vi "clearOrCalcAllPhaseWaveforms_v02.vi"(6 "How Many Experimental Phases?":i32=10 min=1 max=14, 7 "Clear Waveform?":bool, 8 "error in":errorcluster, 9 "Waveform Simulation Jump Filter (Hz)":dbl=100.0, 10 "Waveform Simulation sampling rate (Hz)":i32=1000, 11 "ExperimentOptionsCluster":T1) -> (0 "error out":errorcluster)   [LabVIEW 2019]
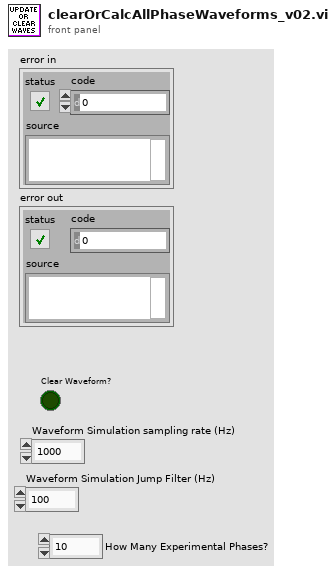
[diagram p1: front panel]
types:
  T1 = cluster{"How Many Experimental Phases?":refnum<vi>, "PhaseA Cluster":cluster{"Phase Experiment Option":refnum<vi>, "Paired Pulse":refnum<vi>, "Jump Train":refnum<vi>, "Voltage Ramp":refnum<vi>, "Voltage Step":refnum<vi>, "Solution Change":refnum<vi>, "Single Jump":refnum<vi>, "Single Manip Jump":refnum<vi>, "Gap Free":refnum<vi>, "Multi Manip Jump":refnum<vi>, "Voltage Pulse":refnum<vi>, "Current Pulse":refnum<vi>, "Current Ramp":refnum<vi>, "Gap Free Iclamp":refnum<vi>}, "PhaseB Cluster":cluster{"Phase Experiment Option":refnum<vi>, "Paired Pulse":refnum<vi>, "Jump Train":refnum<vi>, "Voltage Ramp":refnum<vi>, "Voltage Step":refnum<vi>, "Solution Change":refnum<vi>, "Single Jump":refnum<vi>, "Single Manip Jump":refnum<vi>, "Gap Free":refnum<vi>, "Multi Manip Jump":refnum<vi>, "Voltage Pulse":refnum<vi>, "Current Pulse":refnum<vi>, "Current Ramp":refnum<vi>, "Gap Free Iclamp":refnum<vi>}, "PhaseC Cluster":cluster{"Phase Experiment Option":refnum<vi>, "Paired Pulse":refnum<vi>, "Jump Train":refnum<vi>, "Voltage Ramp":refnum<vi>, "Voltage Step":refnum<vi>, "Solution Change":refnum<vi>, "Single Jump":refnum<vi>, "Single Manip Jump":refnum<vi>, "Gap Free":refnum<vi>, "Multi Manip Jump":refnum<vi>, "Voltage Pulse":refnum<vi>, "Current Pulse":refnum<vi>, "Current Ramp":refnum<vi>, "Gap Free Iclamp":refnum<vi>}, "PhaseD Cluster":cluster{"Phase Experiment Option":refnum<vi>, "Paired Pulse":refnum<vi>, "Jump Train":refnum<vi>, "Voltage Ramp":refnum<vi>, "Voltage Step":refnum<vi>, "Solution Change":refnum<vi>, "Single Jump":refnum<vi>, "Single Manip Jump":refnum<vi>, "Gap Free":refnum<vi>, "Multi Manip Jump":refnum<vi>, "Voltage Pulse":refnum<vi>, "Current Pulse":refnum<vi>, "Current Ramp":refnum<vi>, "Gap Free Iclamp":refnum<vi>}, "PhaseE Cluster":cluster{"Phase Experiment Option":refnum<vi>, "Paired Pulse":refnum<vi>, "Jump Train":refnum<vi>, "Voltage Ramp":refnum<vi>, "Voltage Step":refnum<vi>, "Solution Change":refnum<vi>, "Single Jump":refnum<vi>, "Single Manip Jump":refnum<vi>, "Gap Free":refnum<vi>, "Multi Manip Jump":refnum<vi>, "Voltage Pulse":refnum<vi>, "Current Pulse":refnum<vi>, "Current Ramp":refnum<vi>, "Gap Free Iclamp":refnum<vi>}, "PhaseF Cluster":cluster{"Phase Experiment Option":refnum<vi>, "Paired Pulse":refnum<vi>, "Jump Train":refnum<vi>, "Voltage Ramp":refnum<vi>, "Voltage Step":refnum<vi>, "Solution Change":refnum<vi>, "Single Jump":refnum<vi>, "Single Manip Jump":refnum<vi>, "Gap Free":refnum<vi>, "Multi Manip Jump":refnum<vi>, "Voltage Pulse":refnum<vi>, "Current Pulse":refnum<vi>, "Current Ramp":refnum<vi>, "Gap Free Iclamp":refnum<vi>}, "time to wait for solution change (min)":refnum<vi>, "valve Time Cluster":cluster{"time of Last V1 Change":refnum<vi>, "time of Last V2 Change":refnum<vi>, "time of Last V3 Change":refnum<vi>}, "PhaseG Cluster":cluster{"Phase Experiment Option":refnum<vi>, "Paired Pulse":refnum<vi>, "Jump Train":refnum<vi>, "Voltage Ramp":refnum<vi>, "Voltage Step":refnum<vi>, "Solution Change":refnum<vi>, "Single Jump":refnum<vi>, "Single Manip Jump":refnum<vi>, "Gap Free":refnum<vi>, "Multi Manip Jump":refnum<vi>, "Voltage Pulse":refnum<vi>, "Current Pulse":refnum<vi>, "Current Ramp":refnum<vi>, "Gap Free Iclamp":refnum<vi>}, "PhaseH Cluster":cluster{"Phase Experiment Option":refnum<vi>, "Paired Pulse":refnum<vi>, "Jump Train":refnum<vi>, "Voltage Ramp":refnum<vi>, "Voltage Step":refnum<vi>, "Solution Change":refnum<vi>, "Single Jump":refnum<vi>, "Single Manip Jump":refnum<vi>, "Gap Free":refnum<vi>, "Multi Manip Jump":refnum<vi>, "Voltage Pulse":refnum<vi>, "Current Pulse":refnum<vi>, "Current Ramp":refnum<vi>, "Gap Free Iclamp":refnum<vi>}, "PhaseI Cluster":cluster{"Phase Experiment Option":refnum<vi>, "Paired Pulse":refnum<vi>, "Jump Train":refnum<vi>, "Voltage Ramp":refnum<vi>, "Voltage Step":refnum<vi>, "Solution Change":refnum<vi>, "Single Jump":refnum<vi>, "Single Manip Jump":refnum<vi>, "Gap Free":refnum<vi>, "Multi Manip Jump":refnum<vi>, "Voltage Pulse":refnum<vi>, "Current Pulse":refnum<vi>, "Current Ramp":refnum<vi>, "Gap Free Iclamp":refnum<vi>}, "PhaseJ Cluster":cluster{"Phase Experiment Option":refnum<vi>, "Paired Pulse":refnum<vi>, "Jump Train":refnum<vi>, "Voltage Ramp":refnum<vi>, "Voltage Step":refnum<vi>, "Solution Change":refnum<vi>, "Single Jump":refnum<vi>, "Single Manip Jump":refnum<vi>, "Gap Free":refnum<vi>, "Multi Manip Jump":refnum<vi>, "Voltage Pulse":refnum<vi>, "Current Pulse":refnum<vi>, "Current Ramp":refnum<vi>, "Gap Free Iclamp":refnum<vi>}, "PhaseK Cluster":cluster{"Phase Experiment Option":refnum<vi>, "Paired Pulse":refnum<vi>, "Jump Train":refnum<vi>, "Voltage Ramp":refnum<vi>, "Voltage Step":refnum<vi>, "Solution Change":refnum<vi>, "Single Jump":refnum<vi>, "Single Manip Jump":refnum<vi>, "Gap Free":refnum<vi>, "Multi Manip Jump":refnum<vi>, "Voltage Pulse":refnum<vi>, "Current Pulse":refnum<vi>, "Current Ramp":refnum<vi>, "Gap Free Iclamp":refnum<vi>}, "PhaseL Cluster":cluster{"Phase Experiment Option":refnum<vi>, "Paired Pulse":refnum<vi>, "Jump Train":refnum<vi>, "Voltage Ramp":refnum<vi>, "Voltage Step":refnum<vi>, "Solution Change":refnum<vi>, "Single Jump":refnum<vi>, "Single Manip Jump":refnum<vi>, "Gap Free":refnum<vi>, "Multi Manip Jump":refnum<vi>, "Voltage Pulse":refnum<vi>, "Current Pulse":refnum<vi>, "Current Ramp":refnum<vi>, "Gap Free Iclamp":refnum<vi>}, "PhaseStatusCluster":cluster{"Phase A Done":refnum<vi>, "Phase B Done":refnum<vi>, "Phase C Done":refnum<vi>, "Phase D Done":refnum<vi>, "Phase E Done":refnum<vi>, "Phase F Done":refnum<vi>, "Phase G Done":refnum<vi>, "Phase H Done":refnum<vi>, "Phase I Done":refnum<vi>, "Phase J Done":refnum<vi>, "Phase K Done":refnum<vi>, "Phase L Done":refnum<vi>}}
  T2 = cluster{"Phase Experiment Option":refnum<vi>, "Paired Pulse":refnum<vi>, "Jump Train":refnum<vi>, "Voltage Ramp":refnum<vi>, "Voltage Step":refnum<vi>, "Solution Change":refnum<vi>, "Single Jump":refnum<vi>, "Single Manip Jump":refnum<vi>, "Gap Free":refnum<vi>, "Multi Manip Jump":refnum<vi>, "Voltage Pulse":refnum<vi>, "Current Pulse":refnum<vi>, "Current Ramp":refnum<vi>, "Gap Free Iclamp":refnum<vi>}
  T3 = cluster{"Which Position to use for Experiment":enum16{"Jumper Safe Position", "Experiment Safe Position", "Jumper Position A", "Jumper Position B", "Jumper Position C", "Jumper Position o-A", "Jumper Position A-o", "Jumper Position A-B", "Jumper Position B-A", "Jumper Position B-C", "Jumper Position C-B", "Jumper Position C-o", "Jumper Position o-C", "Don't Move"}, "Start Position (N)":string, "Jump Position (m)":string, "Duration (s)":dbl, "Delay (s)":dbl, "Pulse Width (s)":dbl, "Replicates":dbl, "Pulse Delay (s)":dbl, "Pulse Delta Delay (s)":dbl, "Vholding (mV)":dbl, "Valve 1 Position":i16, "Valve 2 Position":i16, "valve 1 used now?":bool, "valve 2 used now?":bool, "valve 3 used now? ":bool, "Valve 3 Position":i16, "protocol Preview":waveform(dbl)[]}
  T4 = cluster{"Which Position to use for Experiment":enum16{"Jumper Safe Position", "Experiment Safe Position", "Jumper Position A", "Jumper Position B", "Jumper Position C", "Jumper Position o-A", "Jumper Position A-o", "Jumper Position A-B", "Jumper Position B-A", "Jumper Position B-C", "Jumper Position C-B", "Jumper Position C-o", "Jumper Position o-C", "Don't Move"}, "Start Position (N)":string, "Jump Position (m)":string, "Duration (s)":dbl, "Delay (s)":dbl, "Pulse Width (s)":dbl, "Valve 1 Position":i16, "Valve 2 Position":i16, "Replicates":dbl, "Pulse Period (s)":dbl, "Vholding (mV)":dbl, "Number of Pulses":dbl, "valve 1 used now?":bool, "valve 2 used now?":bool, "valve 3 used now? ":bool, "Valve 3 Position":i16, "protocol Preview":waveform(dbl)[]}
  T5 = cluster{"Which Position to use for Experiment":enum16{"Jumper Safe Position", "Experiment Safe Position", "Jumper Position A", "Jumper Position B", "Jumper Position C", "Jumper Position o-A", "Jumper Position A-o", "Jumper Position A-B", "Jumper Position B-A", "Jumper Position B-C", "Jumper Position C-B", "Jumper Position C-o", "Jumper Position o-C", "Don't Move"}, "Duration (s)":dbl, "Delay (s)":dbl, "Ramp Slope (mV/s)":dbl, "Voltage Start (mV)":dbl, "Replicates":dbl, "Voltage End (mV)":dbl, "Ramp Duration (s)":dbl, "Vholding (mV)":dbl, "Valve 1 Position":i16, "Valve 2 Position":i16, "Valve 3 Position":i16, "valve 1 used now?":bool, "valve 2 used now?":bool, "valve 3 used now? ":bool, "Maintain Final Voltage until end?":bool, "protocol Preview":waveform(dbl)[]}
  T6 = cluster{"Which Position to use for Experiment":enum16{"Jumper Safe Position", "Experiment Safe Position", "Jumper Position A", "Jumper Position B", "Jumper Position C", "Jumper Position o-A", "Jumper Position A-o", "Jumper Position A-B", "Jumper Position B-A", "Jumper Position B-C", "Jumper Position C-B", "Jumper Position C-o", "Jumper Position o-C", "Don't Move"}, "Duration (s)":dbl, "Delay (s)":dbl, "Ramp Slope (pA/s)":dbl, "Current Start (pA)":dbl, "Replicates":dbl, "Current End (pA)":dbl, "Ramp Duration (s)":dbl, "Iholding (pA)":dbl, "Valve 1 Position":i16, "Valve 2 Position":i16, "Valve 3 Position":i16, "valve 1 used now?":bool, "valve 2 used now?":bool, "valve 3 used now? ":bool, "Maintain Final Voltage until end?":bool, "protocol Preview":waveform(dbl)[]}
  T7 = cluster{"Which Position to use for Experiment":enum16{"Jumper Safe Position", "Experiment Safe Position", "Jumper Position A", "Jumper Position B", "Jumper Position C", "Jumper Position o-A", "Jumper Position A-o", "Jumper Position A-B", "Jumper Position B-A", "Jumper Position B-C", "Jumper Position C-B", "Jumper Position C-o", "Jumper Position o-C", "Don't Move"}, "Duration (s)":dbl, "Delay (s)":dbl, "Step Width (s)":dbl, "Voltage Start (mV)":dbl, "Voltage Step (mV)":dbl, "Replicates":dbl, "Voltage End (mV)":dbl, "Number of Step":dbl, "Vholding (mV)":dbl, "Valve 1 Position":i16, "Valve 2 Position":i16, "Valve 3 Position":i16, "valve 1 used now?":bool, "valve 2 used now?":bool, "valve 3 used now? ":bool, "Total Step Time (s)":dbl, "Maintain Final Voltage until end?":bool, "protocol Preview":waveform(dbl)[]}
  T8 = cluster{"Which Position to use for Experiment":enum16{"Jumper Safe Position", "Experiment Safe Position", "Jumper Position A", "Jumper Position B", "Jumper Position C", "Jumper Position o-A", "Jumper Position A-o", "Jumper Position A-B", "Jumper Position B-A", "Jumper Position B-C", "Jumper Position C-B", "Jumper Position C-o", "Jumper Position o-C", "Don't Move"}, "Duration (s)":dbl, "Delay (s)":dbl, "Pulse Width (s)":dbl, "Which Valve to Change?":i16, "Valve Jump Position":i16, "Replicates":dbl, "Vholding (mV)":dbl, "valve 1 used now?":bool, "valve 2 used now?":bool, "valve 3 used now? ":bool, "Valve 1 Position":i16, "Valve 2 Position":i16, "Valve 3 Position":i16, "protocol Preview":waveform(dbl)[]}
  T9 = cluster{"Which Position to use for Experiment":enum16{"Jumper Safe Position", "Experiment Safe Position", "Jumper Position A", "Jumper Position B", "Jumper Position C", "Jumper Position o-A", "Jumper Position A-o", "Jumper Position A-B", "Jumper Position B-A", "Jumper Position B-C", "Jumper Position C-B", "Jumper Position C-o", "Jumper Position o-C", "Don't Move"}, "Start Position (N)":string, "Jump Position (m)":string, "Duration (s)":dbl, "Delay (s)":dbl, "Pulse Width (s)":dbl, "Valve 1 Position":i16, "Valve 2 Position":i16, "Replicates":dbl, "Vholding (mV)":dbl, "Valve 3 Position":i16, "valve 1 used now?":bool, "valve 2 used now?":bool, "valve 3 used now? ":bool, "protocol Preview":waveform(dbl)[]}
  T10 = cluster{"Start Position (N)":enum16{"Jumper Safe Position", "Experiment Safe Position", "Jumper Position A", "Jumper Position B", "Jumper Position C", "Jumper Position o-A", "Jumper Position A-o", "Jumper Position A-B", "Jumper Position B-A", "Jumper Position B-C", "Jumper Position C-B", "Jumper Position C-o", "Jumper Position o-C", "Don't Move"}, "Duration (s)":dbl, "Delay (s)":dbl, "Pulse Width (s)":dbl, "Valve 1 Position":i16, "Valve 2 Position":i16, "Replicates":dbl, "Jump Position (m)":enum16{"Jumper Safe Position", "Experiment Safe Position", "Jumper Position A", "Jumper Position B", "Jumper Position C", "Jumper Position o-A", "Jumper Position A-o", "Jumper Position A-B", "Jumper Position B-A", "Jumper Position B-C", "Jumper Position C-B", "Jumper Position C-o", "Jumper Position o-C", "Don't Move"}, "Vholding (mV)":dbl, "Valve 3 Position":i16, "valve 1 used now?":bool, "valve 2 used now?":bool, "valve 3 used now? ":bool, "protocol Preview":waveform(dbl)[]}
  T11 = cluster{"Start Position (N)":enum16{"Jumper Safe Position", "Experiment Safe Position", "Jumper Position A", "Jumper Position B", "Jumper Position C", "Jumper Position o-A", "Jumper Position A-o", "Jumper Position A-B", "Jumper Position B-A", "Jumper Position B-C", "Jumper Position C-B", "Jumper Position C-o", "Jumper Position o-C"}, "Duration (s)":dbl, "Delay (s)":dbl, "Valve 1 Position":i16, "Valve 2 Position":i16, "Replicates":dbl, "Vholding (mV)":dbl, "Valve 3 Position":i16, "valve 1 used now?":bool, "valve 2 used now?":bool, "valve 3 used now? ":bool, "Jump Position Array":enum16{"Jumper Safe Position", "Experiment Safe Position", "Jumper Position A", "Jumper Position B", "Jumper Position C", "Jumper Position o-A", "Jumper Position A-o", "Jumper Position A-B", "Jumper Position B-A", "Jumper Position B-C", "Jumper Position C-B", "Jumper Position C-o", "Jumper Position o-C"}[], "Position Dwell Time (s)":dbl[], "protocol Preview":waveform(dbl)[]}
  T12 = cluster{"Which Position to use for Experiment":enum16{"Jumper Safe Position", "Experiment Safe Position", "Jumper Position A", "Jumper Position B", "Jumper Position C", "Jumper Position o-A", "Jumper Position A-o", "Jumper Position A-B", "Jumper Position B-A", "Jumper Position B-C", "Jumper Position C-B", "Jumper Position C-o", "Jumper Position o-C", "Don't Move"}, "Duration (s)":dbl, "Delay (s)":dbl, "Pulse 2 (s)":dbl, "Pulse 1 (mV)":dbl, "Replicates":dbl, "Pulse 1 (s)":dbl, "Pulse 2 (mV)":dbl, "Vholding (mV)":dbl, "Valve 1 Position":i16, "Valve 2 Position":i16, "Valve 3 Position":i16, "valve 1 used now?":bool, "valve 2 used now?":bool, "valve 3 used now? ":bool, "Maintain Final Voltage until end?":bool, "delta Pulse 1 (mV)":dbl, "delta Pulse 2 (mV)":dbl, "Sweeps":dbl, "Final Pulse 1 (mV)":dbl, "Final Pulse 2 (mV)":dbl, "protocol Preview":waveform(dbl)[]}
  T13 = cluster{"Which Position to use for Experiment":enum16{"Jumper Safe Position", "Experiment Safe Position", "Jumper Position A", "Jumper Position B", "Jumper Position C", "Jumper Position o-A", "Jumper Position A-o", "Jumper Position A-B", "Jumper Position B-A", "Jumper Position B-C", "Jumper Position C-B", "Jumper Position C-o", "Jumper Position o-C", "Don't Move"}, "Duration (s)":dbl, "Delay (s)":dbl, "Pulse 2 (s)":dbl, "Pulse 1 (pA)":dbl, "Replicates":dbl, "Pulse 1 (s)":dbl, "Pulse 2 (pA)":dbl, "Iholding (pA)":dbl, "Valve 1 Position":i16, "Valve 2 Position":i16, "Valve 3 Position":i16, "valve 1 used now?":bool, "valve 2 used now?":bool, "valve 3 used now? ":bool, "Maintain Final Voltage until end?":bool, "delta Pulse 1 (pA)":dbl, "delta Pulse 2 (pA)":dbl, "Sweeps":dbl, "Final Pulse 1 (pA)":dbl, "Final Pulse 2 (pA)":dbl, "protocol Preview":waveform(dbl)[]}
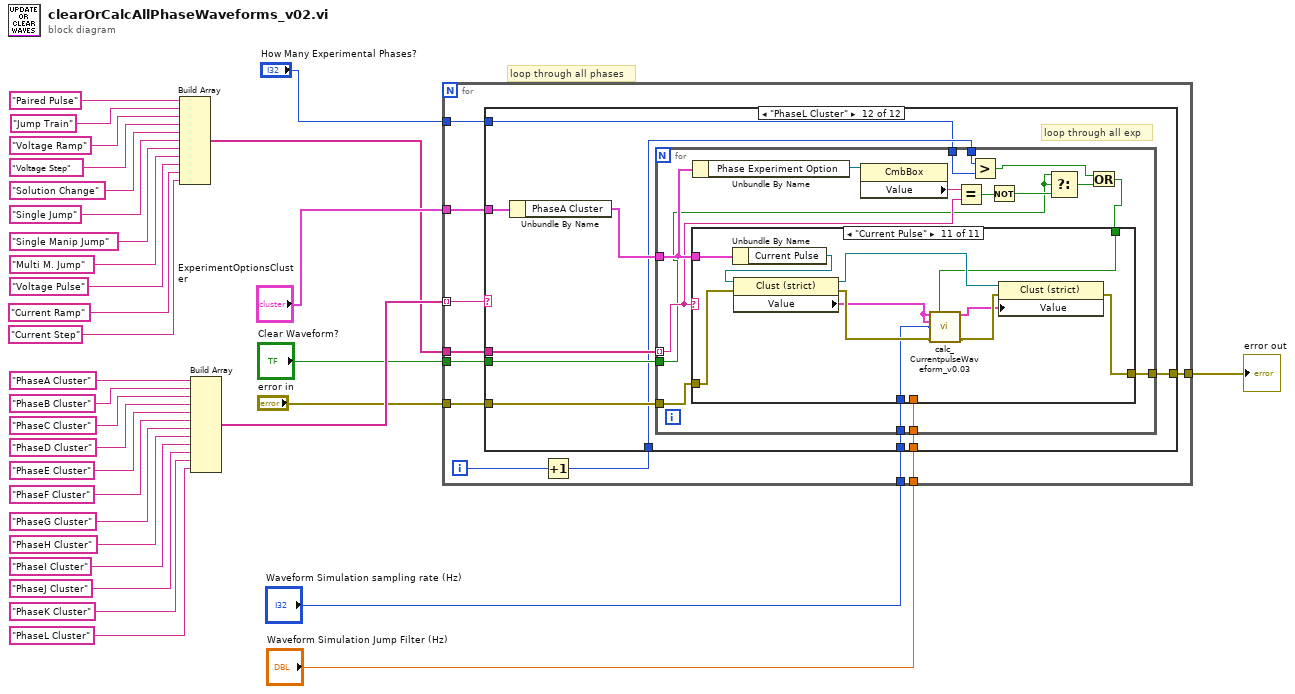
[diagram p0: block diagram]
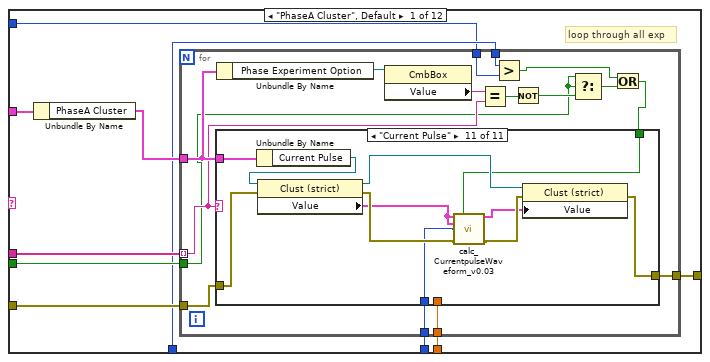
[diagram p2: hidden frame]
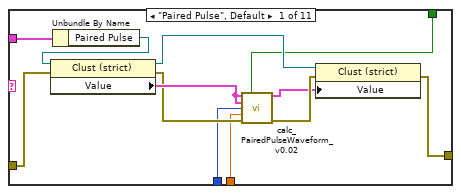
[diagram p3: hidden frame]
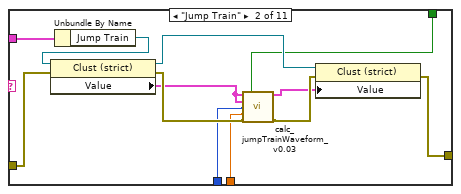
[diagram p4: hidden frame]
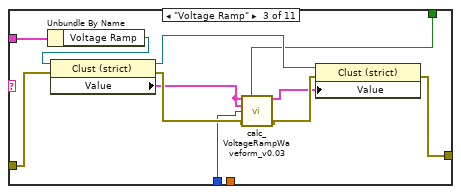
[diagram p5: hidden frame]
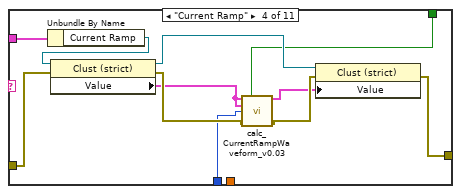
[diagram p6: hidden frame]
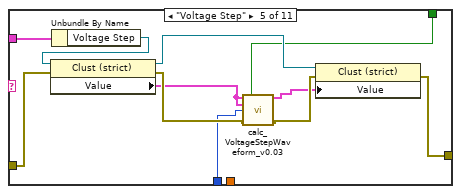
[diagram p7: hidden frame]
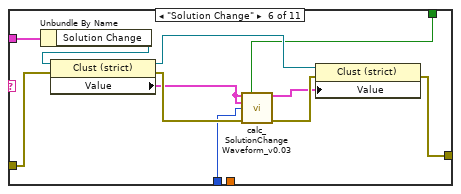
[diagram p8: hidden frame]
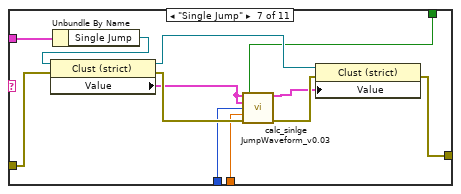
[diagram p9: hidden frame]
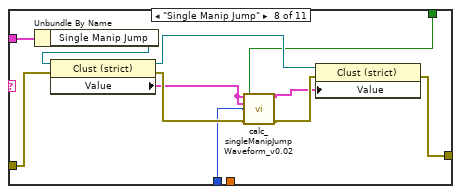
[diagram p10: hidden frame]
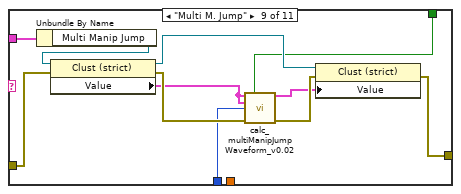
[diagram p11: hidden frame]
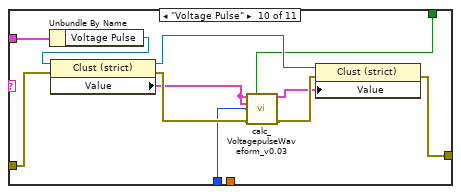
[diagram p12: hidden frame]
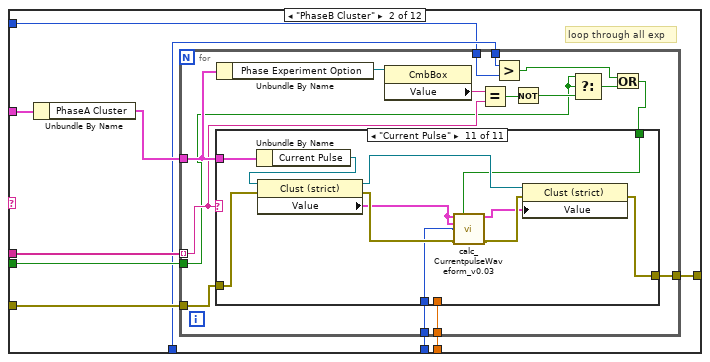
[diagram p13: hidden frame]
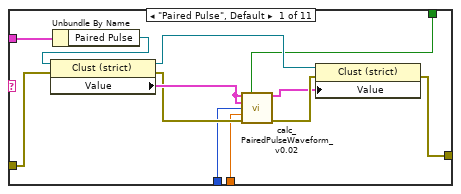
[diagram p14: hidden frame]
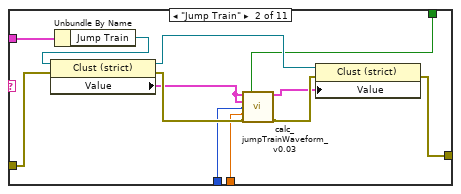
[diagram p15: hidden frame]
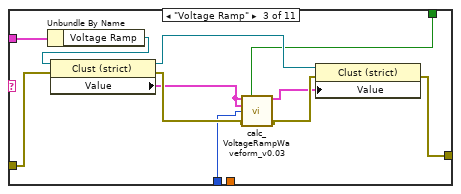
[diagram p16: hidden frame]
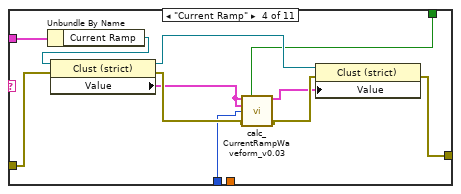
[diagram p17: hidden frame]
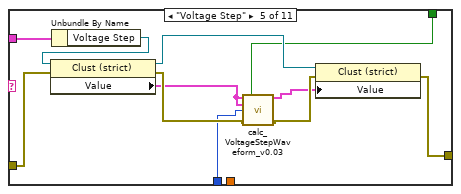
[diagram p18: hidden frame]
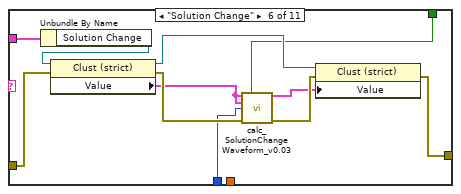
[diagram p19: hidden frame]
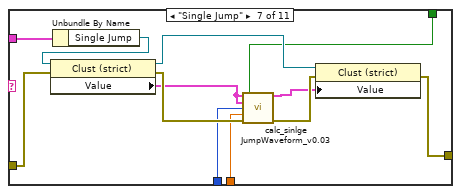
[diagram p20: hidden frame]
diagram:
  # "loop through all phases"
  n1 = Build Array("Paired Pulse", "Jump Train", "Voltage Ramp", "Voltage Step", "Solution Change", "Single Jump", "Single Manip Jump", "Multi M. Jump", "Voltage Pulse", "Current Ramp", "Current Step") -> (w9:string[])
  n2 = Build Array("PhaseA Cluster", "PhaseB Cluster", "PhaseC Cluster", "PhaseD Cluster", "PhaseE Cluster", "PhaseF Cluster", "PhaseG Cluster", "PhaseH Cluster", "PhaseI Cluster", "PhaseJ Cluster", "PhaseK Cluster", "PhaseL Cluster") -> (w19:string[])
  n3 = for {
    tunnel: "ExperimentOptionsCluster" -> [w43]
    tunnel: w19 -> [w42] mode=indexing
    tunnel: w9 -> [w41]
    tunnel: "error in" -> [w40]
    tunnel: [w39] -> w7
    tunnel: "Clear Waveform?" -> [w38]
    tunnel: "Waveform Simulation sampling rate (Hz)" -> [w37]
    tunnel: "Waveform Simulation Jump Filter (Hz)" -> [w36]
    tunnel: "How Many Experimental Phases?" -> [w34]
    i -> [w35]
    n4 = Increment(x=w35) -> (x+1=w33:i32)
    n5 = case shown="\"PhaseL Cluster\"" w42 {
      tunnel: w43 -> [w53 w203 w353 w503 w653 w803 w953 w1103 w1253 w1403 w1553 w1703]
      tunnel: w41 -> [w51 w201 w351 w501 w651 w801 w951 w1101 w1251 w1401 w1551 w1701]
      tunnel: w40 -> [w50 w200 w350 w500 w650 w800 w950 w1100 w1250 w1400 w1550 w1700]
      tunnel: [w49 w199 w349 w499 w649 w799 w949 w1099 w1249 w1399 w1549 w1699] -> w39
      tunnel: w38 -> [w48 w198 w348 w498 w648 w798 w948 w1098 w1248 w1398 w1548 w1698]
      tunnel: w37 -> [w47 w197 w347 w497 w647 w797 w947 w1097 w1247 w1397 w1547 w1697]
      tunnel: w36 -> [w46 w196 w346 w496 w646 w796 w946 w1096 w1246 w1396 w1546 w1696]
      tunnel: w33 -> [w45 w195 w345 w495 w645 w795 w945 w1095 w1245 w1395 w1545 w1695]
      tunnel: w34 -> [w44 w194 w344 w494 w644 w794 w944 w1094 w1244 w1394 w1544 w1694]
      frame "PhaseA Cluster", Default {
        # "loop through all exp"
        n6 = Unbundle By Name(w53) -> ("PhaseA Cluster"=w52:T2)
        n7 = for {
          tunnel: w52 -> [w67]
          tunnel: w51 -> [w64] mode=indexing
          tunnel: w50 -> [w69]
          tunnel: [w68] -> w49
          tunnel: w48 -> [w57]
          tunnel: w47 -> [w63]
          tunnel: w46 -> [w62]
          tunnel: w45 -> [w61]
          tunnel: w44 -> [w60]
          n8 = Unbundle By Name(w67) -> ("Phase Experiment Option"=w66:refnum<vi>)
          n9 = property class="CmbBox"(reference=w66) -> ("Value"=w65:string)  [unwired: 1 in, 2 out]
          n10 = Equal?(x=w65, y=w64) -> (x = y?=w58:bool)
          n11 = Greater?(x=w61, y=w60) -> (0:w55:bool)
          n12 = Not(x=w58) -> (.not. x?=w59:bool)
          n13 = Select(t=w57, s=w57, f=w59) -> (s? t:f=w56:bool)
          n14 = Or(x=w55, y=w56) -> (x .or. y?=w54:bool)
          n15 = case shown="\"Current Pulse\"" w64 {
            tunnel: w67 -> [w81 w93 w104 w115 w126 w137 w149 w160 w171 w182 w193]
            tunnel: w69 -> [w77 w90 w101 w112 w123 w134 w146 w157 w168 w179 w190]
            tunnel: [w74 w89 w100 w111 w122 w133 w145 w156 w167 w178 w189] -> w68
            tunnel: w63 -> [w72 w85 w97 w108 w119 w130 w140 w153 w164 w175 w186]
            tunnel: w62 -> [w71 w86 _ _ _ _ w139 _ _ _ _]
            tunnel: w54 -> [w70 w82 w94 w105 w116 w127 w138 w150 w161 w172 w183]
            frame "Paired Pulse", Default {
              n16 = Unbundle By Name(w81) -> ("Paired Pulse"=w80:refnum<vi>)
              n17 = property class="Clust (strict)"(reference=w80, error in=w77) -> (reference out=w78:refnum<vi>, error out=w76:errorcluster, "Value"=w79:T3)
              n18 = call "calc_PairedPulseWaveform_v0.02.vi"("New input cluster"=w79, "Clear Waveform?"=w70, "Old input cluster"=w79, "Numeric"=w72, "Jump Filter Freq (Hz)"=w71, "error in"=w76) -> ("output cluster"=w73:T3, "error out"=w75:errorcluster)  [unwired: 8 in]
              n19 = property class="Clust (strict)"(reference=w78, error in=w75, "Value"=w73) -> (error out=w74:errorcluster)  [unwired: 1 out]
            }
            frame "Jump Train" {
              n20 = Unbundle By Name(w93) -> ("Jump Train"=w92:refnum<vi>)
              n21 = property class="Clust (strict)"(reference=w92, error in=w90) -> (reference out=w91:refnum<vi>, error out=w88:errorcluster, "Value"=w84:T4)
              n22 = call "calc_jumpTrainWaveform_v0.03.vi"("New input cluster"=w84, "Clear Waveform?"=w82, "Old input cluster"=w84, "sample freq"=w85, "Jump Filter Freq (Hz)"=w86, "error in"=w88) -> ("output cluster"=w83:T4, "error out"=w87:errorcluster)  [unwired: 8 in]
              n23 = property class="Clust (strict)"(reference=w91, error in=w87, "Value"=w83) -> (error out=w89:errorcluster)  [unwired: 1 out]
            }
            frame "Voltage Ramp" {
              n24 = Unbundle By Name(w104) -> ("Voltage Ramp"=w103:refnum<vi>)
              n25 = property class="Clust (strict)"(reference=w103, error in=w101) -> (reference out=w102:refnum<vi>, error out=w98:errorcluster, "Value"=w96:T5)
              n26 = call "calc_VoltageRampWaveform_v0.03.vi"("New input cluster"=w96, "Clear Waveform?"=w94, "Old input cluster"=w96, "sample freq"=w97, "error in"=w98) -> ("output cluster"=w95:T5, "error out"=w99:errorcluster)  [unwired: 9 in]
              n27 = property class="Clust (strict)"(reference=w102, error in=w99, "Value"=w95) -> (error out=w100:errorcluster)  [unwired: 1 out]
            }
            frame "Current Ramp" {
              n28 = Unbundle By Name(w115) -> ("Current Ramp"=w114:refnum<vi>)
              n29 = property class="Clust (strict)"(reference=w114, error in=w112) -> (reference out=w113:refnum<vi>, error out=w109:errorcluster, "Value"=w107:T6)
              n30 = call "calc_CurrentRampWaveform_v0.03.vi"("New input cluster"=w107, "Clear Waveform?"=w105, "Old input cluster"=w107, "sample freq"=w108, "error in"=w109) -> ("output cluster"=w106:T6, "error out"=w110:errorcluster)  [unwired: 9 in]
              n31 = property class="Clust (strict)"(reference=w113, error in=w110, "Value"=w106) -> (error out=w111:errorcluster)  [unwired: 1 out]
            }
            frame "Voltage Step" {
              n32 = Unbundle By Name(w126) -> ("Voltage Step"=w125:refnum<vi>)
              n33 = property class="Clust (strict)"(reference=w125, error in=w123) -> (reference out=w124:refnum<vi>, error out=w120:errorcluster, "Value"=w118:T7)
              n34 = call "calc_VoltageStepWaveform_v0.03.vi"("New input cluster"=w118, "Clear Waveform?"=w116, "Old input cluster"=w118, "sample freq"=w119, "error in"=w120) -> ("output cluster"=w117:T7, "error out"=w121:errorcluster)  [unwired: 9 in]
              n35 = property class="Clust (strict)"(reference=w124, error in=w121, "Value"=w117) -> (error out=w122:errorcluster)  [unwired: 1 out]
            }
            frame "Solution Change" {
              n36 = Unbundle By Name(w137) -> ("Solution Change"=w136:refnum<vi>)
              n37 = property class="Clust (strict)"(reference=w136, error in=w134) -> (reference out=w135:refnum<vi>, error out=w131:errorcluster, "Value"=w129:T8)
              n38 = call "calc_SolutionChangeWaveform_v0.03.vi"("New input cluster"=w129, "Clear Waveform?"=w127, "Old input cluster"=w129, "sample freq"=w130, "error in"=w131) -> ("output cluster"=w128:T8, "error out"=w132:errorcluster)  [unwired: 9 in]
              n39 = property class="Clust (strict)"(reference=w135, error in=w132, "Value"=w128) -> (error out=w133:errorcluster)  [unwired: 1 out]
            }
            frame "Single Jump" {
              n40 = Unbundle By Name(w149) -> ("Single Jump"=w148:refnum<vi>)
              n41 = property class="Clust (strict)"(reference=w148, error in=w146) -> (reference out=w147:refnum<vi>, error out=w144:errorcluster, "Value"=w141:T9)
              n42 = call "calc_sinlge JumpWaveform_v0.03.vi"("New input cluster"=w141, "Clear Waveform?"=w138, "Old input cluster"=w141, "sample freq"=w140, "Jump Filter Freq (Hz)"=w139, "error in"=w144) -> ("output cluster"=w142:T9, "error out"=w143:errorcluster)  [unwired: 8 in]
              n43 = property class="Clust (strict)"(reference=w147, error in=w143, "Value"=w142) -> (error out=w145:errorcluster)  [unwired: 1 out]
            }
            frame "Single Manip Jump" {
              n44 = Unbundle By Name(w160) -> ("Single Manip Jump"=w159:refnum<vi>)
              n45 = property class="Clust (strict)"(reference=w159, error in=w157) -> (reference out=w158:refnum<vi>, error out=w154:errorcluster, "Value"=w152:T10)
              n46 = call "calc_singleManipJumpWaveform_v0.02.vi"("New input cluster"=w152, "Clear Waveform?"=w150, "Old input cluster"=w152, "simulate Wave freq"=w153, "error in"=w154) -> ("output cluster"=w151:T10, "error out"=w155:errorcluster)  [unwired: 9 in]
              n47 = property class="Clust (strict)"(reference=w158, error in=w155, "Value"=w151) -> (error out=w156:errorcluster)  [unwired: 1 out]
            }
            frame "Multi M. Jump" {
              n48 = Unbundle By Name(w171) -> ("Multi Manip Jump"=w170:refnum<vi>)
              n49 = property class="Clust (strict)"(reference=w170, error in=w168) -> (reference out=w169:refnum<vi>, error out=w165:errorcluster, "Value"=w163:T11)
              n50 = call "calc_multiManipJumpWaveform_v0.02.vi"("New input cluster"=w163, "Clear Waveform?"=w161, "Old input cluster"=w163, "Numeric"=w164, "error in"=w165) -> ("output cluster"=w162:T11, "error out"=w166:errorcluster)  [unwired: 9 in]
              n51 = property class="Clust (strict)"(reference=w169, error in=w166, "Value"=w162) -> (error out=w167:errorcluster)  [unwired: 1 out]
            }
            frame "Voltage Pulse" {
              n52 = Unbundle By Name(w182) -> ("Voltage Pulse"=w181:refnum<vi>)
              n53 = property class="Clust (strict)"(reference=w181, error in=w179) -> (reference out=w180:refnum<vi>, error out=w176:errorcluster, "Value"=w174:T12)
              n54 = call "calc_VoltagepulseWaveform_v0.03.vi"("New input cluster"=w174, "Clear Waveform?"=w172, "Old input cluster"=w174, "sample freq"=w175, "error in"=w176) -> ("output cluster"=w173:T12, "error out"=w177:errorcluster)  [unwired: 9 in]
              n55 = property class="Clust (strict)"(reference=w180, error in=w177, "Value"=w173) -> (error out=w178:errorcluster)  [unwired: 1 out]
            }
            frame "Current Pulse" {
              n56 = Unbundle By Name(w193) -> ("Current Pulse"=w192:refnum<vi>)
              n57 = property class="Clust (strict)"(reference=w192, error in=w190) -> (reference out=w191:refnum<vi>, error out=w187:errorcluster, "Value"=w185:T13)
              n58 = call "calc_CurrentpulseWaveform_v0.03.vi"("New input cluster"=w185, "Clear Waveform?"=w183, "Old input cluster"=w185, "sample freq"=w186, "error in"=w187) -> ("output cluster"=w184:T13, "error out"=w188:errorcluster)  [unwired: 9 in]
              n59 = property class="Clust (strict)"(reference=w191, error in=w188, "Value"=w184) -> (error out=w189:errorcluster)  [unwired: 1 out]
            }
          }
        }
      }
      frame "PhaseB Cluster" {
        # "loop through all exp"
        n60 = Unbundle By Name(w203) -> ("PhaseA Cluster"=w202:T2)
        n61 = for {
          tunnel: w202 -> [w217]
          tunnel: w201 -> [w214] mode=indexing
          tunnel: w200 -> [w219]
          tunnel: [w218] -> w199
          tunnel: w198 -> [w207]
          tunnel: w197 -> [w213]
          tunnel: w196 -> [w212]
          tunnel: w195 -> [w211]
          tunnel: w194 -> [w210]
          n62 = Unbundle By Name(w217) -> ("Phase Experiment Option"=w216:refnum<vi>)
          n63 = property class="CmbBox"(reference=w216) -> ("Value"=w215:string)  [unwired: 1 in, 2 out]
          n64 = Equal?(x=w215, y=w214) -> (x = y?=w208:bool)
          n65 = Greater?(x=w211, y=w210) -> (0:w205:bool)
          n66 = Not(x=w208) -> (.not. x?=w209:bool)
          n67 = Select(t=w207, s=w207, f=w209) -> (s? t:f=w206:bool)
          n68 = Or(x=w205, y=w206) -> (x .or. y?=w204:bool)
          n69 = case shown="\"Current Pulse\"" w214 {
            tunnel: w217 -> [w231 w243 w254 w265 w276 w287 w299 w310 w321 w332 w343]
            tunnel: w219 -> [w227 w240 w251 w262 w273 w284 w296 w307 w318 w329 w340]
            tunnel: [w224 w239 w250 w261 w272 w283 w295 w306 w317 w328 w339] -> w218
            tunnel: w213 -> [w222 w235 w247 w258 w269 w280 w290 w303 w314 w325 w336]
            tunnel: w212 -> [w221 w236 _ _ _ _ w289 _ _ _ _]
            tunnel: w204 -> [w220 w232 w244 w255 w266 w277 w288 w300 w311 w322 w333]
            frame "Paired Pulse", Default {
              n70 = Unbundle By Name(w231) -> ("Paired Pulse"=w230:refnum<vi>)
              n71 = property class="Clust (strict)"(reference=w230, error in=w227) -> (reference out=w228:refnum<vi>, error out=w226:errorcluster, "Value"=w229:T3)
              n72 = call "calc_PairedPulseWaveform_v0.02.vi"("New input cluster"=w229, "Clear Waveform?"=w220, "Old input cluster"=w229, "Numeric"=w222, "Jump Filter Freq (Hz)"=w221, "error in"=w226) -> ("output cluster"=w223:T3, "error out"=w225:errorcluster)  [unwired: 8 in]
              n73 = property class="Clust (strict)"(reference=w228, error in=w225, "Value"=w223) -> (error out=w224:errorcluster)  [unwired: 1 out]
            }
            frame "Jump Train" {
              n74 = Unbundle By Name(w243) -> ("Jump Train"=w242:refnum<vi>)
              n75 = property class="Clust (strict)"(reference=w242, error in=w240) -> (reference out=w241:refnum<vi>, error out=w238:errorcluster, "Value"=w234:T4)
              n76 = call "calc_jumpTrainWaveform_v0.03.vi"("New input cluster"=w234, "Clear Waveform?"=w232, "Old input cluster"=w234, "sample freq"=w235, "Jump Filter Freq (Hz)"=w236, "error in"=w238) -> ("output cluster"=w233:T4, "error out"=w237:errorcluster)  [unwired: 8 in]
              n77 = property class="Clust (strict)"(reference=w241, error in=w237, "Value"=w233) -> (error out=w239:errorcluster)  [unwired: 1 out]
            }
            frame "Voltage Ramp" {
              n78 = Unbundle By Name(w254) -> ("Voltage Ramp"=w253:refnum<vi>)
              n79 = property class="Clust (strict)"(reference=w253, error in=w251) -> (reference out=w252:refnum<vi>, error out=w248:errorcluster, "Value"=w246:T5)
              n80 = call "calc_VoltageRampWaveform_v0.03.vi"("New input cluster"=w246, "Clear Waveform?"=w244, "Old input cluster"=w246, "sample freq"=w247, "error in"=w248) -> ("output cluster"=w245:T5, "error out"=w249:errorcluster)  [unwired: 9 in]
              n81 = property class="Clust (strict)"(reference=w252, error in=w249, "Value"=w245) -> (error out=w250:errorcluster)  [unwired: 1 out]
            }
            frame "Current Ramp" {
              n82 = Unbundle By Name(w265) -> ("Current Ramp"=w264:refnum<vi>)
              n83 = property class="Clust (strict)"(reference=w264, error in=w262) -> (reference out=w263:refnum<vi>, error out=w259:errorcluster, "Value"=w257:T6)
              n84 = call "calc_CurrentRampWaveform_v0.03.vi"("New input cluster"=w257, "Clear Waveform?"=w255, "Old input cluster"=w257, "sample freq"=w258, "error in"=w259) -> ("output cluster"=w256:T6, "error out"=w260:errorcluster)  [unwired: 9 in]
              n85 = property class="Clust (strict)"(reference=w263, error in=w260, "Value"=w256) -> (error out=w261:errorcluster)  [unwired: 1 out]
            }
            frame "Voltage Step" {
              n86 = Unbundle By Name(w276) -> ("Voltage Step"=w275:refnum<vi>)
              n87 = property class="Clust (strict)"(reference=w275, error in=w273) -> (reference out=w274:refnum<vi>, error out=w270:errorcluster, "Value"=w268:T7)
              n88 = call "calc_VoltageStepWaveform_v0.03.vi"("New input cluster"=w268, "Clear Waveform?"=w266, "Old input cluster"=w268, "sample freq"=w269, "error in"=w270) -> ("output cluster"=w267:T7, "error out"=w271:errorcluster)  [unwired: 9 in]
              n89 = property class="Clust (strict)"(reference=w274, error in=w271, "Value"=w267) -> (error out=w272:errorcluster)  [unwired: 1 out]
            }
            frame "Solution Change" {
              n90 = Unbundle By Name(w287) -> ("Solution Change"=w286:refnum<vi>)
              n91 = property class="Clust (strict)"(reference=w286, error in=w284) -> (reference out=w285:refnum<vi>, error out=w281:errorcluster, "Value"=w279:T8)
              n92 = call "calc_SolutionChangeWaveform_v0.03.vi"("New input cluster"=w279, "Clear Waveform?"=w277, "Old input cluster"=w279, "sample freq"=w280, "error in"=w281) -> ("output cluster"=w278:T8, "error out"=w282:errorcluster)  [unwired: 9 in]
              n93 = property class="Clust (strict)"(reference=w285, error in=w282, "Value"=w278) -> (error out=w283:errorcluster)  [unwired: 1 out]
            }
            frame "Single Jump" {
              n94 = Unbundle By Name(w299) -> ("Single Jump"=w298:refnum<vi>)
              n95 = property class="Clust (strict)"(reference=w298, error in=w296) -> (reference out=w297:refnum<vi>, error out=w294:errorcluster, "Value"=w291:T9)
              n96 = call "calc_sinlge JumpWaveform_v0.03.vi"("New input cluster"=w291, "Clear Waveform?"=w288, "Old input cluster"=w291, "sample freq"=w290, "Jump Filter Freq (Hz)"=w289, "error in"=w294) -> ("output cluster"=w292:T9, "error out"=w293:errorcluster)  [unwired: 8 in]
              n97 = property class="Clust (strict)"(reference=w297, error in=w293, "Value"=w292) -> (error out=w295:errorcluster)  [unwired: 1 out]
            }
            frame "Single Manip Jump" {
              n98 = Unbundle By Name(w310) -> ("Single Manip Jump"=w309:refnum<vi>)
              n99 = property class="Clust (strict)"(reference=w309, error in=w307) -> (reference out=w308:refnum<vi>, error out=w304:errorcluster, "Value"=w302:T10)
              n100 = call "calc_singleManipJumpWaveform_v0.02.vi"("New input cluster"=w302, "Clear Waveform?"=w300, "Old input cluster"=w302, "simulate Wave freq"=w303, "error in"=w304) -> ("output cluster"=w301:T10, "error out"=w305:errorcluster)  [unwired: 9 in]
              n101 = property class="Clust (strict)"(reference=w308, error in=w305, "Value"=w301) -> (error out=w306:errorcluster)  [unwired: 1 out]
            }
            frame "Multi M. Jump" {
              n102 = Unbundle By Name(w321) -> ("Multi Manip Jump"=w320:refnum<vi>)
              n103 = property class="Clust (strict)"(reference=w320, error in=w318) -> (reference out=w319:refnum<vi>, error out=w315:errorcluster, "Value"=w313:T11)
              n104 = call "calc_multiManipJumpWaveform_v0.02.vi"("New input cluster"=w313, "Clear Waveform?"=w311, "Old input cluster"=w313, "Numeric"=w314, "error in"=w315) -> ("output cluster"=w312:T11, "error out"=w316:errorcluster)  [unwired: 9 in]
              n105 = property class="Clust (strict)"(reference=w319, error in=w316, "Value"=w312) -> (error out=w317:errorcluster)  [unwired: 1 out]
            }
            frame "Voltage Pulse" {
              n106 = Unbundle By Name(w332) -> ("Voltage Pulse"=w331:refnum<vi>)
              n107 = property class="Clust (strict)"(reference=w331, error in=w329) -> (reference out=w330:refnum<vi>, error out=w326:errorcluster, "Value"=w324:T12)
              n108 = call "calc_VoltagepulseWaveform_v0.03.vi"("New input cluster"=w324, "Clear Waveform?"=w322, "Old input cluster"=w324, "sample freq"=w325, "error in"=w326) -> ("output cluster"=w323:T12, "error out"=w327:errorcluster)  [unwired: 9 in]
              n109 = property class="Clust (strict)"(reference=w330, error in=w327, "Value"=w323) -> (error out=w328:errorcluster)  [unwired: 1 out]
            }
            frame "Current Pulse" {
              n110 = Unbundle By Name(w343) -> ("Current Pulse"=w342:refnum<vi>)
              n111 = property class="Clust (strict)"(reference=w342, error in=w340) -> (reference out=w341:refnum<vi>, error out=w337:errorcluster, "Value"=w335:T13)
              n112 = call "calc_CurrentpulseWaveform_v0.03.vi"("New input cluster"=w335, "Clear Waveform?"=w333, "Old input cluster"=w335, "sample freq"=w336, "error in"=w337) -> ("output cluster"=w334:T13, "error out"=w338:errorcluster)  [unwired: 9 in]
              n113 = property class="Clust (strict)"(reference=w341, error in=w338, "Value"=w334) -> (error out=w339:errorcluster)  [unwired: 1 out]
            }
          }
        }
      }
      frame "PhaseC Cluster" {
        # "loop through all exp"
        n114 = Unbundle By Name(w353) -> ("PhaseA Cluster"=w352:T2)
        n115 = for {
          tunnel: w352 -> [w367]
          tunnel: w351 -> [w364] mode=indexing
          tunnel: w350 -> [w369]
          tunnel: [w368] -> w349
          tunnel: w348 -> [w357]
          tunnel: w347 -> [w363]
          tunnel: w346 -> [w362]
          tunnel: w345 -> [w361]
          tunnel: w344 -> [w360]
          n116 = Unbundle By Name(w367) -> ("Phase Experiment Option"=w366:refnum<vi>)
          n117 = property class="CmbBox"(reference=w366) -> ("Value"=w365:string)  [unwired: 1 in, 2 out]
          n118 = Equal?(x=w365, y=w364) -> (x = y?=w358:bool)
          n119 = Greater?(x=w361, y=w360) -> (0:w355:bool)
          n120 = Not(x=w358) -> (.not. x?=w359:bool)
          n121 = Select(t=w357, s=w357, f=w359) -> (s? t:f=w356:bool)
          n122 = Or(x=w355, y=w356) -> (x .or. y?=w354:bool)
          n123 = case shown="\"Current Pulse\"" w364 {
            tunnel: w367 -> [w381 w393 w404 w415 w426 w437 w449 w460 w471 w482 w493]
            tunnel: w369 -> [w377 w390 w401 w412 w423 w434 w446 w457 w468 w479 w490]
            tunnel: [w374 w389 w400 w411 w422 w433 w445 w456 w467 w478 w489] -> w368
            tunnel: w363 -> [w372 w385 w397 w408 w419 w430 w440 w453 w464 w475 w486]
            tunnel: w362 -> [w371 w386 _ _ _ _ w439 _ _ _ _]
            tunnel: w354 -> [w370 w382 w394 w405 w416 w427 w438 w450 w461 w472 w483]
            frame "Paired Pulse", Default {
              n124 = Unbundle By Name(w381) -> ("Paired Pulse"=w380:refnum<vi>)
              n125 = property class="Clust (strict)"(reference=w380, error in=w377) -> (reference out=w378:refnum<vi>, error out=w376:errorcluster, "Value"=w379:T3)
              n126 = call "calc_PairedPulseWaveform_v0.02.vi"("New input cluster"=w379, "Clear Waveform?"=w370, "Old input cluster"=w379, "Numeric"=w372, "Jump Filter Freq (Hz)"=w371, "error in"=w376) -> ("output cluster"=w373:T3, "error out"=w375:errorcluster)  [unwired: 8 in]
              n127 = property class="Clust (strict)"(reference=w378, error in=w375, "Value"=w373) -> (error out=w374:errorcluster)  [unwired: 1 out]
            }
            frame "Jump Train" {
              n128 = Unbundle By Name(w393) -> ("Jump Train"=w392:refnum<vi>)
              n129 = property class="Clust (strict)"(reference=w392, error in=w390) -> (reference out=w391:refnum<vi>, error out=w388:errorcluster, "Value"=w384:T4)
              n130 = call "calc_jumpTrainWaveform_v0.03.vi"("New input cluster"=w384, "Clear Waveform?"=w382, "Old input cluster"=w384, "sample freq"=w385, "Jump Filter Freq (Hz)"=w386, "error in"=w388) -> ("output cluster"=w383:T4, "error out"=w387:errorcluster)  [unwired: 8 in]
              n131 = property class="Clust (strict)"(reference=w391, error in=w387, "Value"=w383) -> (error out=w389:errorcluster)  [unwired: 1 out]
            }
            frame "Voltage Ramp" {
              n132 = Unbundle By Name(w404) -> ("Voltage Ramp"=w403:refnum<vi>)
              n133 = property class="Clust (strict)"(reference=w403, error in=w401) -> (reference out=w402:refnum<vi>, error out=w398:errorcluster, "Value"=w396:T5)
              n134 = call "calc_VoltageRampWaveform_v0.03.vi"("New input cluster"=w396, "Clear Waveform?"=w394, "Old input cluster"=w396, "sample freq"=w397, "error in"=w398) -> ("output cluster"=w395:T5, "error out"=w399:errorcluster)  [unwired: 9 in]
              n135 = property class="Clust (strict)"(reference=w402, error in=w399, "Value"=w395) -> (error out=w400:errorcluster)  [unwired: 1 out]
            }
            frame "Current Ramp" {
              n136 = Unbundle By Name(w415) -> ("Current Ramp"=w414:refnum<vi>)
              n137 = property class="Clust (strict)"(reference=w414, error in=w412) -> (reference out=w413:refnum<vi>, error out=w409:errorcluster, "Value"=w407:T6)
              n138 = call "calc_CurrentRampWaveform_v0.03.vi"("New input cluster"=w407, "Clear Waveform?"=w405, "Old input cluster"=w407, "sample freq"=w408, "error in"=w409) -> ("output cluster"=w406:T6, "error out"=w410:errorcluster)  [unwired: 9 in]
              n139 = property class="Clust (strict)"(reference=w413, error in=w410, "Value"=w406) -> (error out=w411:errorcluster)  [unwired: 1 out]
            }
            frame "Voltage Step" {
              n140 = Unbundle By Name(w426) -> ("Voltage Step"=w425:refnum<vi>)
              n141 = property class="Clust (strict)"(reference=w425, error in=w423) -> (reference out=w424:refnum<vi>, error out=w420:errorcluster, "Value"=w418:T7)
              n142 = call "calc_VoltageStepWaveform_v0.03.vi"("New input cluster"=w418, "Clear Waveform?"=w416, "Old input cluster"=w418, "sample freq"=w419, "error in"=w420) -> ("output cluster"=w417:T7, "error out"=w421:errorcluster)  [unwired: 9 in]
              n143 = property class="Clust (strict)"(reference=w424, error in=w421, "Value"=w417) -> (error out=w422:errorcluster)  [unwired: 1 out]
            }
            frame "Solution Change" {
              n144 = Unbundle By Name(w437) -> ("Solution Change"=w436:refnum<vi>)
              n145 = property class="Clust (strict)"(reference=w436, error in=w434) -> (reference out=w435:refnum<vi>, error out=w431:errorcluster, "Value"=w429:T8)
              n146 = call "calc_SolutionChangeWaveform_v0.03.vi"("New input cluster"=w429, "Clear Waveform?"=w427, "Old input cluster"=w429, "sample freq"=w430, "error in"=w431) -> ("output cluster"=w428:T8, "error out"=w432:errorcluster)  [unwired: 9 in]
              n147 = property class="Clust (strict)"(reference=w435, error in=w432, "Value"=w428) -> (error out=w433:errorcluster)  [unwired: 1 out]
            }
            frame "Single Jump" {
              n148 = Unbundle By Name(w449) -> ("Single Jump"=w448:refnum<vi>)
              n149 = property class="Clust (strict)"(reference=w448, error in=w446) -> (reference out=w447:refnum<vi>, error out=w444:errorcluster, "Value"=w441:T9)
              n150 = call "calc_sinlge JumpWaveform_v0.03.vi"("New input cluster"=w441, "Clear Waveform?"=w438, "Old input cluster"=w441, "sample freq"=w440, "Jump Filter Freq (Hz)"=w439, "error in"=w444) -> ("output cluster"=w442:T9, "error out"=w443:errorcluster)  [unwired: 8 in]
              n151 = property class="Clust (strict)"(reference=w447, error in=w443, "Value"=w442) -> (error out=w445:errorcluster)  [unwired: 1 out]
            }
            frame "Single Manip Jump" {
              n152 = Unbundle By Name(w460) -> ("Single Manip Jump"=w459:refnum<vi>)
              n153 = property class="Clust (strict)"(reference=w459, error in=w457) -> (reference out=w458:refnum<vi>, error out=w454:errorcluster, "Value"=w452:T10)
              n154 = call "calc_singleManipJumpWaveform_v0.02.vi"("New input cluster"=w452, "Clear Waveform?"=w450, "Old input cluster"=w452, "simulate Wave freq"=w453, "error in"=w454) -> ("output cluster"=w451:T10, "error out"=w455:errorcluster)  [unwired: 9 in]
              n155 = property class="Clust (strict)"(reference=w458, error in=w455, "Value"=w451) -> (error out=w456:errorcluster)  [unwired: 1 out]
            }
            frame "Multi M. Jump" {
              n156 = Unbundle By Name(w471) -> ("Multi Manip Jump"=w470:refnum<vi>)
              n157 = property class="Clust (strict)"(reference=w470, error in=w468) -> (reference out=w469:refnum<vi>, error out=w465:errorcluster, "Value"=w463:T11)
              n158 = call "calc_multiManipJumpWaveform_v0.02.vi"("New input cluster"=w463, "Clear Waveform?"=w461, "Old input cluster"=w463, "Numeric"=w464, "error in"=w465) -> ("output cluster"=w462:T11, "error out"=w466:errorcluster)  [unwired: 9 in]
              n159 = property class="Clust (strict)"(reference=w469, error in=w466, "Value"=w462) -> (error out=w467:errorcluster)  [unwired: 1 out]
            }
            frame "Voltage Pulse" {
              n160 = Unbundle By Name(w482) -> ("Voltage Pulse"=w481:refnum<vi>)
              n161 = property class="Clust (strict)"(reference=w481, error in=w479) -> (reference out=w480:refnum<vi>, error out=w476:errorcluster, "Value"=w474:T12)
              n162 = call "calc_VoltagepulseWaveform_v0.03.vi"("New input cluster"=w474, "Clear Waveform?"=w472, "Old input cluster"=w474, "sample freq"=w475, "error in"=w476) -> ("output cluster"=w473:T12, "error out"=w477:errorcluster)  [unwired: 9 in]
              n163 = property class="Clust (strict)"(reference=w480, error in=w477, "Value"=w473) -> (error out=w478:errorcluster)  [unwired: 1 out]
            }
            frame "Current Pulse" {
              n164 = Unbundle By Name(w493) -> ("Current Pulse"=w492:refnum<vi>)
              n165 = property class="Clust (strict)"(reference=w492, error in=w490) -> (reference out=w491:refnum<vi>, error out=w487:errorcluster, "Value"=w485:T13)
              n166 = call "calc_CurrentpulseWaveform_v0.03.vi"("New input cluster"=w485, "Clear Waveform?"=w483, "Old input cluster"=w485, "sample freq"=w486, "error in"=w487) -> ("output cluster"=w484:T13, "error out"=w488:errorcluster)  [unwired: 9 in]
              n167 = property class="Clust (strict)"(reference=w491, error in=w488, "Value"=w484) -> (error out=w489:errorcluster)  [unwired: 1 out]
            }
          }
        }
      }
      frame "PhaseD Cluster" {
        # "loop through all exp"
        n168 = Unbundle By Name(w503) -> ("PhaseA Cluster"=w502:T2)
        n169 = for {
          tunnel: w502 -> [w517]
          tunnel: w501 -> [w514] mode=indexing
          tunnel: w500 -> [w519]
          tunnel: [w518] -> w499
          tunnel: w498 -> [w507]
          tunnel: w497 -> [w513]
          tunnel: w496 -> [w512]
          tunnel: w495 -> [w511]
          tunnel: w494 -> [w510]
          n170 = Unbundle By Name(w517) -> ("Phase Experiment Option"=w516:refnum<vi>)
          n171 = property class="CmbBox"(reference=w516) -> ("Value"=w515:string)  [unwired: 1 in, 2 out]
          n172 = Equal?(x=w515, y=w514) -> (x = y?=w508:bool)
          n173 = Greater?(x=w511, y=w510) -> (0:w505:bool)
          n174 = Not(x=w508) -> (.not. x?=w509:bool)
          n175 = Select(t=w507, s=w507, f=w509) -> (s? t:f=w506:bool)
          n176 = Or(x=w505, y=w506) -> (x .or. y?=w504:bool)
          n177 = case shown="\"Current Pulse\"" w514 {
            tunnel: w517 -> [w531 w543 w554 w565 w576 w587 w599 w610 w621 w632 w643]
            tunnel: w519 -> [w527 w540 w551 w562 w573 w584 w596 w607 w618 w629 w640]
            tunnel: [w524 w539 w550 w561 w572 w583 w595 w606 w617 w628 w639] -> w518
            tunnel: w513 -> [w522 w535 w547 w558 w569 w580 w590 w603 w614 w625 w636]
            tunnel: w512 -> [w521 w536 _ _ _ _ w589 _ _ _ _]
            tunnel: w504 -> [w520 w532 w544 w555 w566 w577 w588 w600 w611 w622 w633]
            frame "Paired Pulse", Default {
              n178 = Unbundle By Name(w531) -> ("Paired Pulse"=w530:refnum<vi>)
              n179 = property class="Clust (strict)"(reference=w530, error in=w527) -> (reference out=w528:refnum<vi>, error out=w526:errorcluster, "Value"=w529:T3)
              n180 = call "calc_PairedPulseWaveform_v0.02.vi"("New input cluster"=w529, "Clear Waveform?"=w520, "Old input cluster"=w529, "Numeric"=w522, "Jump Filter Freq (Hz)"=w521, "error in"=w526) -> ("output cluster"=w523:T3, "error out"=w525:errorcluster)  [unwired: 8 in]
              n181 = property class="Clust (strict)"(reference=w528, error in=w525, "Value"=w523) -> (error out=w524:errorcluster)  [unwired: 1 out]
            }
            frame "Jump Train" {
              n182 = Unbundle By Name(w543) -> ("Jump Train"=w542:refnum<vi>)
              n183 = property class="Clust (strict)"(reference=w542, error in=w540) -> (reference out=w541:refnum<vi>, error out=w538:errorcluster, "Value"=w534:T4)
              n184 = call "calc_jumpTrainWaveform_v0.03.vi"("New input cluster"=w534, "Clear Waveform?"=w532, "Old input cluster"=w534, "sample freq"=w535, "Jump Filter Freq (Hz)"=w536, "error in"=w538) -> ("output cluster"=w533:T4, "error out"=w537:errorcluster)  [unwired: 8 in]
              n185 = property class="Clust (strict)"(reference=w541, error in=w537, "Value"=w533) -> (error out=w539:errorcluster)  [unwired: 1 out]
            }
            frame "Voltage Ramp" {
              n186 = Unbundle By Name(w554) -> ("Voltage Ramp"=w553:refnum<vi>)
              n187 = property class="Clust (strict)"(reference=w553, error in=w551) -> (reference out=w552:refnum<vi>, error out=w548:errorcluster, "Value"=w546:T5)
              n188 = call "calc_VoltageRampWaveform_v0.03.vi"("New input cluster"=w546, "Clear Waveform?"=w544, "Old input cluster"=w546, "sample freq"=w547, "error in"=w548) -> ("output cluster"=w545:T5, "error out"=w549:errorcluster)  [unwired: 9 in]
              n189 = property class="Clust (strict)"(reference=w552, error in=w549, "Value"=w545) -> (error out=w550:errorcluster)  [unwired: 1 out]
            }
            frame "Current Ramp" {
              n190 = Unbundle By Name(w565) -> ("Current Ramp"=w564:refnum<vi>)
              n191 = property class="Clust (strict)"(reference=w564, error in=w562) -> (reference out=w563:refnum<vi>, error out=w559:errorcluster, "Value"=w557:T6)
              n192 = call "calc_CurrentRampWaveform_v0.03.vi"("New input cluster"=w557, "Clear Waveform?"=w555, "Old input cluster"=w557, "sample freq"=w558, "error in"=w559) -> ("output cluster"=w556:T6, "error out"=w560:errorcluster)  [unwired: 9 in]
              n193 = property class="Clust (strict)"(reference=w563, error in=w560, "Value"=w556) -> (error out=w561:errorcluster)  [unwired: 1 out]
            }
            frame "Voltage Step" {
              n194 = Unbundle By Name(w576) -> ("Voltage Step"=w575:refnum<vi>)
              n195 = property class="Clust (strict)"(reference=w575, error in=w573) -> (reference out=w574:refnum<vi>, error out=w570:errorcluster, "Value"=w568:T7)
              n196 = call "calc_VoltageStepWaveform_v0.03.vi"("New input cluster"=w568, "Clear Waveform?"=w566, "Old input cluster"=w568, "sample freq"=w569, "error in"=w570) -> ("output cluster"=w567:T7, "error out"=w571:errorcluster)  [unwired: 9 in]
              n197 = property class="Clust (strict)"(reference=w574, error in=w571, "Value"=w567) -> (error out=w572:errorcluster)  [unwired: 1 out]
            }
            frame "Solution Change" {
              n198 = Unbundle By Name(w587) -> ("Solution Change"=w586:refnum<vi>)
              n199 = property class="Clust (strict)"(reference=w586, error in=w584) -> (reference out=w585:refnum<vi>, error out=w581:errorcluster, "Value"=w579:T8)
              n200 = call "calc_SolutionChangeWaveform_v0.03.vi"("New input cluster"=w579, "Clear Waveform?"=w577, "Old input cluster"=w579, "sample freq"=w580, "error in"=w581) -> ("output cluster"=w578:T8, "error out"=w582:errorcluster)  [unwired: 9 in]
              n201 = property class="Clust (strict)"(reference=w585, error in=w582, "Value"=w578) -> (error out=w583:errorcluster)  [unwired: 1 out]
            }
            frame "Single Jump" {
              n202 = Unbundle By Name(w599) -> ("Single Jump"=w598:refnum<vi>)
              n203 = property class="Clust (strict)"(reference=w598, error in=w596) -> (reference out=w597:refnum<vi>, error out=w594:errorcluster, "Value"=w591:T9)
              n204 = call "calc_sinlge JumpWaveform_v0.03.vi"("New input cluster"=w591, "Clear Waveform?"=w588, "Old input cluster"=w591, "sample freq"=w590, "Jump Filter Freq (Hz)"=w589, "error in"=w594) -> ("output cluster"=w592:T9, "error out"=w593:errorcluster)  [unwired: 8 in]
              n205 = property class="Clust (strict)"(reference=w597, error in=w593, "Value"=w592) -> (error out=w595:errorcluster)  [unwired: 1 out]
            }
            frame "Single Manip Jump" {
              n206 = Unbundle By Name(w610) -> ("Single Manip Jump"=w609:refnum<vi>)
              n207 = property class="Clust (strict)"(reference=w609, error in=w607) -> (reference out=w608:refnum<vi>, error out=w604:errorcluster, "Value"=w602:T10)
              n208 = call "calc_singleManipJumpWaveform_v0.02.vi"("New input cluster"=w602, "Clear Waveform?"=w600, "Old input cluster"=w602, "simulate Wave freq"=w603, "error in"=w604) -> ("output cluster"=w601:T10, "error out"=w605:errorcluster)  [unwired: 9 in]
              n209 = property class="Clust (strict)"(reference=w608, error in=w605, "Value"=w601) -> (error out=w606:errorcluster)  [unwired: 1 out]
            }
            frame "Multi M. Jump" {
              n210 = Unbundle By Name(w621) -> ("Multi Manip Jump"=w620:refnum<vi>)
              n211 = property class="Clust (strict)"(reference=w620, error in=w618) -> (reference out=w619:refnum<vi>, error out=w615:errorcluster, "Value"=w613:T11)
              n212 = call "calc_multiManipJumpWaveform_v0.02.vi"("New input cluster"=w613, "Clear Waveform?"=w611, "Old input cluster"=w613, "Numeric"=w614, "error in"=w615) -> ("output cluster"=w612:T11, "error out"=w616:errorcluster)  [unwired: 9 in]
              n213 = property class="Clust (strict)"(reference=w619, error in=w616, "Value"=w612) -> (error out=w617:errorcluster)  [unwired: 1 out]
            }
            frame "Voltage Pulse" {
              n214 = Unbundle By Name(w632) -> ("Voltage Pulse"=w631:refnum<vi>)
              n215 = property class="Clust (strict)"(reference=w631, error in=w629) -> (reference out=w630:refnum<vi>, error out=w626:errorcluster, "Value"=w624:T12)
              n216 = call "calc_VoltagepulseWaveform_v0.03.vi"("New input cluster"=w624, "Clear Waveform?"=w622, "Old input cluster"=w624, "sample freq"=w625, "error in"=w626) -> ("output cluster"=w623:T12, "error out"=w627:errorcluster)  [unwired: 9 in]
              n217 = property class="Clust (strict)"(reference=w630, error in=w627, "Value"=w623) -> (error out=w628:errorcluster)  [unwired: 1 out]
            }
            frame "Current Pulse" {
              n218 = Unbundle By Name(w643) -> ("Current Pulse"=w642:refnum<vi>)
              n219 = property class="Clust (strict)"(reference=w642, error in=w640) -> (reference out=w641:refnum<vi>, error out=w637:errorcluster, "Value"=w635:T13)
              n220 = call "calc_CurrentpulseWaveform_v0.03.vi"("New input cluster"=w635, "Clear Waveform?"=w633, "Old input cluster"=w635, "sample freq"=w636, "error in"=w637) -> ("output cluster"=w634:T13, "error out"=w638:errorcluster)  [unwired: 9 in]
              n221 = property class="Clust (strict)"(reference=w641, error in=w638, "Value"=w634) -> (error out=w639:errorcluster)  [unwired: 1 out]
            }
          }
        }
      }
      frame "PhaseE Cluster" {
        # "loop through all exp"
        n222 = Unbundle By Name(w653) -> ("PhaseA Cluster"=w652:T2)
        n223 = for {
          tunnel: w652 -> [w667]
          tunnel: w651 -> [w664] mode=indexing
          tunnel: w650 -> [w669]
          tunnel: [w668] -> w649
          tunnel: w648 -> [w657]
          tunnel: w647 -> [w663]
          tunnel: w646 -> [w662]
          tunnel: w645 -> [w661]
          tunnel: w644 -> [w660]
          n224 = Unbundle By Name(w667) -> ("Phase Experiment Option"=w666:refnum<vi>)
          n225 = property class="CmbBox"(reference=w666) -> ("Value"=w665:string)  [unwired: 1 in, 2 out]
          n226 = Equal?(x=w665, y=w664) -> (x = y?=w658:bool)
          n227 = Greater?(x=w661, y=w660) -> (0:w655:bool)
          n228 = Not(x=w658) -> (.not. x?=w659:bool)
          n229 = Select(t=w657, s=w657, f=w659) -> (s? t:f=w656:bool)
          n230 = Or(x=w655, y=w656) -> (x .or. y?=w654:bool)
          n231 = case shown="\"Current Pulse\"" w664 {
            tunnel: w667 -> [w681 w693 w704 w715 w726 w737 w749 w760 w771 w782 w793]
            tunnel: w669 -> [w677 w690 w701 w712 w723 w734 w746 w757 w768 w779 w790]
            tunnel: [w674 w689 w700 w711 w722 w733 w745 w756 w767 w778 w789] -> w668
            tunnel: w663 -> [w672 w685 w697 w708 w719 w730 w740 w753 w764 w775 w786]
            tunnel: w662 -> [w671 w686 _ _ _ _ w739 _ _ _ _]
            tunnel: w654 -> [w670 w682 w694 w705 w716 w727 w738 w750 w761 w772 w783]
            frame "Paired Pulse", Default {
              n232 = Unbundle By Name(w681) -> ("Paired Pulse"=w680:refnum<vi>)
              n233 = property class="Clust (strict)"(reference=w680, error in=w677) -> (reference out=w678:refnum<vi>, error out=w676:errorcluster, "Value"=w679:T3)
              n234 = call "calc_PairedPulseWaveform_v0.02.vi"("New input cluster"=w679, "Clear Waveform?"=w670, "Old input cluster"=w679, "Numeric"=w672, "Jump Filter Freq (Hz)"=w671, "error in"=w676) -> ("output cluster"=w673:T3, "error out"=w675:errorcluster)  [unwired: 8 in]
              n235 = property class="Clust (strict)"(reference=w678, error in=w675, "Value"=w673) -> (error out=w674:errorcluster)  [unwired: 1 out]
            }
            frame "Jump Train" {
              n236 = Unbundle By Name(w693) -> ("Jump Train"=w692:refnum<vi>)
              n237 = property class="Clust (strict)"(reference=w692, error in=w690) -> (reference out=w691:refnum<vi>, error out=w688:errorcluster, "Value"=w684:T4)
              n238 = call "calc_jumpTrainWaveform_v0.03.vi"("New input cluster"=w684, "Clear Waveform?"=w682, "Old input cluster"=w684, "sample freq"=w685, "Jump Filter Freq (Hz)"=w686, "error in"=w688) -> ("output cluster"=w683:T4, "error out"=w687:errorcluster)  [unwired: 8 in]
              n239 = property class="Clust (strict)"(reference=w691, error in=w687, "Value"=w683) -> (error out=w689:errorcluster)  [unwired: 1 out]
            }
            frame "Voltage Ramp" {
              n240 = Unbundle By Name(w704) -> ("Voltage Ramp"=w703:refnum<vi>)
              n241 = property class="Clust (strict)"(reference=w703, error in=w701) -> (reference out=w702:refnum<vi>, error out=w698:errorcluster, "Value"=w696:T5)
              n242 = call "calc_VoltageRampWaveform_v0.03.vi"("New input cluster"=w696, "Clear Waveform?"=w694, "Old input cluster"=w696, "sample freq"=w697, "error in"=w698) -> ("output cluster"=w695:T5, "error out"=w699:errorcluster)  [unwired: 9 in]
              n243 = property class="Clust (strict)"(reference=w702, error in=w699, "Value"=w695) -> (error out=w700:errorcluster)  [unwired: 1 out]
            }
            frame "Current Ramp" {
              n244 = Unbundle By Name(w715) -> ("Current Ramp"=w714:refnum<vi>)
              n245 = property class="Clust (strict)"(reference=w714, error in=w712) -> (reference out=w713:refnum<vi>, error out=w709:errorcluster, "Value"=w707:T6)
              n246 = call "calc_CurrentRampWaveform_v0.03.vi"("New input cluster"=w707, "Clear Waveform?"=w705, "Old input cluster"=w707, "sample freq"=w708, "error in"=w709) -> ("output cluster"=w706:T6, "error out"=w710:errorcluster)  [unwired: 9 in]
              n247 = property class="Clust (strict)"(reference=w713, error in=w710, "Value"=w706) -> (error out=w711:errorcluster)  [unwired: 1 out]
            }
            frame "Voltage Step" {
              n248 = Unbundle By Name(w726) -> ("Voltage Step"=w725:refnum<vi>)
              n249 = property class="Clust (strict)"(reference=w725, error in=w723) -> (reference out=w724:refnum<vi>, error out=w720:errorcluster, "Value"=w718:T7)
              n250 = call "calc_VoltageStepWaveform_v0.03.vi"("New input cluster"=w718, "Clear Waveform?"=w716, "Old input cluster"=w718, "sample freq"=w719, "error in"=w720) -> ("output cluster"=w717:T7, "error out"=w721:errorcluster)  [unwired: 9 in]
              n251 = property class="Clust (strict)"(reference=w724, error in=w721, "Value"=w717) -> (error out=w722:errorcluster)  [unwired: 1 out]
            }
            frame "Solution Change" {
              n252 = Unbundle By Name(w737) -> ("Solution Change"=w736:refnum<vi>)
              n253 = property class="Clust (strict)"(reference=w736, error in=w734) -> (reference out=w735:refnum<vi>, error out=w731:errorcluster, "Value"=w729:T8)
              n254 = call "calc_SolutionChangeWaveform_v0.03.vi"("New input cluster"=w729, "Clear Waveform?"=w727, "Old input cluster"=w729, "sample freq"=w730, "error in"=w731) -> ("output cluster"=w728:T8, "error out"=w732:errorcluster)  [unwired: 9 in]
              n255 = property class="Clust (strict)"(reference=w735, error in=w732, "Value"=w728) -> (error out=w733:errorcluster)  [unwired: 1 out]
            }
            frame "Single Jump" {
              n256 = Unbundle By Name(w749) -> ("Single Jump"=w748:refnum<vi>)
              n257 = property class="Clust (strict)"(reference=w748, error in=w746) -> (reference out=w747:refnum<vi>, error out=w744:errorcluster, "Value"=w741:T9)
              n258 = call "calc_sinlge JumpWaveform_v0.03.vi"("New input cluster"=w741, "Clear Waveform?"=w738, "Old input cluster"=w741, "sample freq"=w740, "Jump Filter Freq (Hz)"=w739, "error in"=w744) -> ("output cluster"=w742:T9, "error out"=w743:errorcluster)  [unwired: 8 in]
              n259 = property class="Clust (strict)"(reference=w747, error in=w743, "Value"=w742) -> (error out=w745:errorcluster)  [unwired: 1 out]
            }
            frame "Single Manip Jump" {
              n260 = Unbundle By Name(w760) -> ("Single Manip Jump"=w759:refnum<vi>)
              n261 = property class="Clust (strict)"(reference=w759, error in=w757) -> (reference out=w758:refnum<vi>, error out=w754:errorcluster, "Value"=w752:T10)
              n262 = call "calc_singleManipJumpWaveform_v0.02.vi"("New input cluster"=w752, "Clear Waveform?"=w750, "Old input cluster"=w752, "simulate Wave freq"=w753, "error in"=w754) -> ("output cluster"=w751:T10, "error out"=w755:errorcluster)  [unwired: 9 in]
              n263 = property class="Clust (strict)"(reference=w758, error in=w755, "Value"=w751) -> (error out=w756:errorcluster)  [unwired: 1 out]
            }
            frame "Multi M. Jump" {
              n264 = Unbundle By Name(w771) -> ("Multi Manip Jump"=w770:refnum<vi>)
              n265 = property class="Clust (strict)"(reference=w770, error in=w768) -> (reference out=w769:refnum<vi>, error out=w765:errorcluster, "Value"=w763:T11)
              n266 = call "calc_multiManipJumpWaveform_v0.02.vi"("New input cluster"=w763, "Clear Waveform?"=w761, "Old input cluster"=w763, "Numeric"=w764, "error in"=w765) -> ("output cluster"=w762:T11, "error out"=w766:errorcluster)  [unwired: 9 in]
              n267 = property class="Clust (strict)"(reference=w769, error in=w766, "Value"=w762) -> (error out=w767:errorcluster)  [unwired: 1 out]
            }
            frame "Voltage Pulse" {
              n268 = Unbundle By Name(w782) -> ("Voltage Pulse"=w781:refnum<vi>)
              n269 = property class="Clust (strict)"(reference=w781, error in=w779) -> (reference out=w780:refnum<vi>, error out=w776:errorcluster, "Value"=w774:T12)
              n270 = call "calc_VoltagepulseWaveform_v0.03.vi"("New input cluster"=w774, "Clear Waveform?"=w772, "Old input cluster"=w774, "sample freq"=w775, "error in"=w776) -> ("output cluster"=w773:T12, "error out"=w777:errorcluster)  [unwired: 9 in]
              n271 = property class="Clust (strict)"(reference=w780, error in=w777, "Value"=w773) -> (error out=w778:errorcluster)  [unwired: 1 out]
            }
            frame "Current Pulse" {
              n272 = Unbundle By Name(w793) -> ("Current Pulse"=w792:refnum<vi>)
              n273 = property class="Clust (strict)"(reference=w792, error in=w790) -> (reference out=w791:refnum<vi>, error out=w787:errorcluster, "Value"=w785:T13)
              n274 = call "calc_CurrentpulseWaveform_v0.03.vi"("New input cluster"=w785, "Clear Waveform?"=w783, "Old input cluster"=w785, "sample freq"=w786, "error in"=w787) -> ("output cluster"=w784:T13, "error out"=w788:errorcluster)  [unwired: 9 in]
              n275 = property class="Clust (strict)"(reference=w791, error in=w788, "Value"=w784) -> (error out=w789:errorcluster)  [unwired: 1 out]
            }
          }
        }
      }
      frame "PhaseF Cluster" {
        # "loop through all exp"
        n276 = Unbundle By Name(w803) -> ("PhaseA Cluster"=w802:T2)
        n277 = for {
          tunnel: w802 -> [w817]
          tunnel: w801 -> [w814] mode=indexing
          tunnel: w800 -> [w819]
          tunnel: [w818] -> w799
          tunnel: w798 -> [w807]
          tunnel: w797 -> [w813]
          tunnel: w796 -> [w812]
          tunnel: w795 -> [w811]
          tunnel: w794 -> [w810]
          n278 = Unbundle By Name(w817) -> ("Phase Experiment Option"=w816:refnum<vi>)
          n279 = property class="CmbBox"(reference=w816) -> ("Value"=w815:string)  [unwired: 1 in, 2 out]
          n280 = Equal?(x=w815, y=w814) -> (x = y?=w808:bool)
          n281 = Greater?(x=w811, y=w810) -> (0:w805:bool)
          n282 = Not(x=w808) -> (.not. x?=w809:bool)
          n283 = Select(t=w807, s=w807, f=w809) -> (s? t:f=w806:bool)
          n284 = Or(x=w805, y=w806) -> (x .or. y?=w804:bool)
          n285 = case shown="\"Current Pulse\"" w814 {
            tunnel: w817 -> [w831 w843 w854 w865 w876 w887 w899 w910 w921 w932 w943]
            tunnel: w819 -> [w827 w840 w851 w862 w873 w884 w896 w907 w918 w929 w940]
            tunnel: [w824 w839 w850 w861 w872 w883 w895 w906 w917 w928 w939] -> w818
            tunnel: w813 -> [w822 w835 w847 w858 w869 w880 w890 w903 w914 w925 w936]
            tunnel: w812 -> [w821 w836 _ _ _ _ w889 _ _ _ _]
            tunnel: w804 -> [w820 w832 w844 w855 w866 w877 w888 w900 w911 w922 w933]
            frame "Paired Pulse", Default {
              n286 = Unbundle By Name(w831) -> ("Paired Pulse"=w830:refnum<vi>)
              n287 = property class="Clust (strict)"(reference=w830, error in=w827) -> (reference out=w828:refnum<vi>, error out=w826:errorcluster, "Value"=w829:T3)
              n288 = call "calc_PairedPulseWaveform_v0.02.vi"("New input cluster"=w829, "Clear Waveform?"=w820, "Old input cluster"=w829, "Numeric"=w822, "Jump Filter Freq (Hz)"=w821, "error in"=w826) -> ("output cluster"=w823:T3, "error out"=w825:errorcluster)  [unwired: 8 in]
              n289 = property class="Clust (strict)"(reference=w828, error in=w825, "Value"=w823) -> (error out=w824:errorcluster)  [unwired: 1 out]
            }
            frame "Jump Train" {
              n290 = Unbundle By Name(w843) -> ("Jump Train"=w842:refnum<vi>)
              n291 = property class="Clust (strict)"(reference=w842, error in=w840) -> (reference out=w841:refnum<vi>, error out=w838:errorcluster, "Value"=w834:T4)
              n292 = call "calc_jumpTrainWaveform_v0.03.vi"("New input cluster"=w834, "Clear Waveform?"=w832, "Old input cluster"=w834, "sample freq"=w835, "Jump Filter Freq (Hz)"=w836, "error in"=w838) -> ("output cluster"=w833:T4, "error out"=w837:errorcluster)  [unwired: 8 in]
              n293 = property class="Clust (strict)"(reference=w841, error in=w837, "Value"=w833) -> (error out=w839:errorcluster)  [unwired: 1 out]
            }
            frame "Voltage Ramp" {
              n294 = Unbundle By Name(w854) -> ("Voltage Ramp"=w853:refnum<vi>)
              n295 = property class="Clust (strict)"(reference=w853, error in=w851) -> (reference out=w852:refnum<vi>, error out=w848:errorcluster, "Value"=w846:T5)
              n296 = call "calc_VoltageRampWaveform_v0.03.vi"("New input cluster"=w846, "Clear Waveform?"=w844, "Old input cluster"=w846, "sample freq"=w847, "error in"=w848) -> ("output cluster"=w845:T5, "error out"=w849:errorcluster)  [unwired: 9 in]
              n297 = property class="Clust (strict)"(reference=w852, error in=w849, "Value"=w845) -> (error out=w850:errorcluster)  [unwired: 1 out]
            }
            frame "Current Ramp" {
              n298 = Unbundle By Name(w865) -> ("Current Ramp"=w864:refnum<vi>)
              n299 = property class="Clust (strict)"(reference=w864, error in=w862) -> (reference out=w863:refnum<vi>, error out=w859:errorcluster, "Value"=w857:T6)
              n300 = call "calc_CurrentRampWaveform_v0.03.vi"("New input cluster"=w857, "Clear Waveform?"=w855, "Old input cluster"=w857, "sample freq"=w858, "error in"=w859) -> ("output cluster"=w856:T6, "error out"=w860:errorcluster)  [unwired: 9 in]
              n301 = property class="Clust (strict)"(reference=w863, error in=w860, "Value"=w856) -> (error out=w861:errorcluster)  [unwired: 1 out]
            }
            frame "Voltage Step" {
              n302 = Unbundle By Name(w876) -> ("Voltage Step"=w875:refnum<vi>)
              n303 = property class="Clust (strict)"(reference=w875, error in=w873) -> (reference out=w874:refnum<vi>, error out=w870:errorcluster, "Value"=w868:T7)
              n304 = call "calc_VoltageStepWaveform_v0.03.vi"("New input cluster"=w868, "Clear Waveform?"=w866, "Old input cluster"=w868, "sample freq"=w869, "error in"=w870) -> ("output cluster"=w867:T7, "error out"=w871:errorcluster)  [unwired: 9 in]
              n305 = property class="Clust (strict)"(reference=w874, error in=w871, "Value"=w867) -> (error out=w872:errorcluster)  [unwired: 1 out]
            }
            frame "Solution Change" {
              n306 = Unbundle By Name(w887) -> ("Solution Change"=w886:refnum<vi>)
              n307 = property class="Clust (strict)"(reference=w886, error in=w884) -> (reference out=w885:refnum<vi>, error out=w881:errorcluster, "Value"=w879:T8)
              n308 = call "calc_SolutionChangeWaveform_v0.03.vi"("New input cluster"=w879, "Clear Waveform?"=w877, "Old input cluster"=w879, "sample freq"=w880, "error in"=w881) -> ("output cluster"=w878:T8, "error out"=w882:errorcluster)  [unwired: 9 in]
              n309 = property class="Clust (strict)"(reference=w885, error in=w882, "Value"=w878) -> (error out=w883:errorcluster)  [unwired: 1 out]
            }
            frame "Single Jump" {
              n310 = Unbundle By Name(w899) -> ("Single Jump"=w898:refnum<vi>)
              n311 = property class="Clust (strict)"(reference=w898, error in=w896) -> (reference out=w897:refnum<vi>, error out=w894:errorcluster, "Value"=w891:T9)
              n312 = call "calc_sinlge JumpWaveform_v0.03.vi"("New input cluster"=w891, "Clear Waveform?"=w888, "Old input cluster"=w891, "sample freq"=w890, "Jump Filter Freq (Hz)"=w889, "error in"=w894) -> ("output cluster"=w892:T9, "error out"=w893:errorcluster)  [unwired: 8 in]
              n313 = property class="Clust (strict)"(reference=w897, error in=w893, "Value"=w892) -> (error out=w895:errorcluster)  [unwired: 1 out]
            }
            frame "Single Manip Jump" {
              n314 = Unbundle By Name(w910) -> ("Single Manip Jump"=w909:refnum<vi>)
              n315 = property class="Clust (strict)"(reference=w909, error in=w907) -> (reference out=w908:refnum<vi>, error out=w904:errorcluster, "Value"=w902:T10)
              n316 = call "calc_singleManipJumpWaveform_v0.02.vi"("New input cluster"=w902, "Clear Waveform?"=w900, "Old input cluster"=w902, "simulate Wave freq"=w903, "error in"=w904) -> ("output cluster"=w901:T10, "error out"=w905:errorcluster)  [unwired: 9 in]
              n317 = property class="Clust (strict)"(reference=w908, error in=w905, "Value"=w901) -> (error out=w906:errorcluster)  [unwired: 1 out]
            }
            frame "Multi M. Jump" {
              n318 = Unbundle By Name(w921) -> ("Multi Manip Jump"=w920:refnum<vi>)
              n319 = property class="Clust (strict)"(reference=w920, error in=w918) -> (reference out=w919:refnum<vi>, error out=w915:errorcluster, "Value"=w913:T11)
              n320 = call "calc_multiManipJumpWaveform_v0.02.vi"("New input cluster"=w913, "Clear Waveform?"=w911, "Old input cluster"=w913, "Numeric"=w914, "error in"=w915) -> ("output cluster"=w912:T11, "error out"=w916:errorcluster)  [unwired: 9 in]
              n321 = property class="Clust (strict)"(reference=w919, error in=w916, "Value"=w912) -> (error out=w917:errorcluster)  [unwired: 1 out]
            }
            frame "Voltage Pulse" {
              n322 = Unbundle By Name(w932) -> ("Voltage Pulse"=w931:refnum<vi>)
              n323 = property class="Clust (strict)"(reference=w931, error in=w929) -> (reference out=w930:refnum<vi>, error out=w926:errorcluster, "Value"=w924:T12)
              n324 = call "calc_VoltagepulseWaveform_v0.03.vi"("New input cluster"=w924, "Clear Waveform?"=w922, "Old input cluster"=w924, "sample freq"=w925, "error in"=w926) -> ("output cluster"=w923:T12, "error out"=w927:errorcluster)  [unwired: 9 in]
              n325 = property class="Clust (strict)"(reference=w930, error in=w927, "Value"=w923) -> (error out=w928:errorcluster)  [unwired: 1 out]
            }
            frame "Current Pulse" {
              n326 = Unbundle By Name(w943) -> ("Current Pulse"=w942:refnum<vi>)
              n327 = property class="Clust (strict)"(reference=w942, error in=w940) -> (reference out=w941:refnum<vi>, error out=w937:errorcluster, "Value"=w935:T13)
              n328 = call "calc_CurrentpulseWaveform_v0.03.vi"("New input cluster"=w935, "Clear Waveform?"=w933, "Old input cluster"=w935, "sample freq"=w936, "error in"=w937) -> ("output cluster"=w934:T13, "error out"=w938:errorcluster)  [unwired: 9 in]
              n329 = property class="Clust (strict)"(reference=w941, error in=w938, "Value"=w934) -> (error out=w939:errorcluster)  [unwired: 1 out]
            }
          }
        }
      }
      frame "PhaseG Cluster" {
        # "loop through all exp"
        n330 = Unbundle By Name(w953) -> ("PhaseA Cluster"=w952:T2)
        n331 = for {
          tunnel: w952 -> [w967]
          tunnel: w951 -> [w964] mode=indexing
          tunnel: w950 -> [w969]
          tunnel: [w968] -> w949
          tunnel: w948 -> [w957]
          tunnel: w947 -> [w963]
          tunnel: w946 -> [w962]
          tunnel: w945 -> [w961]
          tunnel: w944 -> [w960]
          n332 = Unbundle By Name(w967) -> ("Phase Experiment Option"=w966:refnum<vi>)
          n333 = property class="CmbBox"(reference=w966) -> ("Value"=w965:string)  [unwired: 1 in, 2 out]
          n334 = Equal?(x=w965, y=w964) -> (x = y?=w958:bool)
          n335 = Greater?(x=w961, y=w960) -> (0:w955:bool)
          n336 = Not(x=w958) -> (.not. x?=w959:bool)
          n337 = Select(t=w957, s=w957, f=w959) -> (s? t:f=w956:bool)
          n338 = Or(x=w955, y=w956) -> (x .or. y?=w954:bool)
          n339 = case shown="\"Current Pulse\"" w964 {
            tunnel: w967 -> [w981 w993 w1004 w1015 w1026 w1037 w1049 w1060 w1071 w1082 w1093]
            tunnel: w969 -> [w977 w990 w1001 w1012 w1023 w1034 w1046 w1057 w1068 w1079 w1090]
            tunnel: [w974 w989 w1000 w1011 w1022 w1033 w1045 w1056 w1067 w1078 w1089] -> w968
            tunnel: w963 -> [w972 w985 w997 w1008 w1019 w1030 w1040 w1053 w1064 w1075 w1086]
            tunnel: w962 -> [w971 w986 _ _ _ _ w1039 _ _ _ _]
            tunnel: w954 -> [w970 w982 w994 w1005 w1016 w1027 w1038 w1050 w1061 w1072 w1083]
            frame "Paired Pulse", Default {
              n340 = Unbundle By Name(w981) -> ("Paired Pulse"=w980:refnum<vi>)
              n341 = property class="Clust (strict)"(reference=w980, error in=w977) -> (reference out=w978:refnum<vi>, error out=w976:errorcluster, "Value"=w979:T3)
              n342 = call "calc_PairedPulseWaveform_v0.02.vi"("New input cluster"=w979, "Clear Waveform?"=w970, "Old input cluster"=w979, "Numeric"=w972, "Jump Filter Freq (Hz)"=w971, "error in"=w976) -> ("output cluster"=w973:T3, "error out"=w975:errorcluster)  [unwired: 8 in]
              n343 = property class="Clust (strict)"(reference=w978, error in=w975, "Value"=w973) -> (error out=w974:errorcluster)  [unwired: 1 out]
            }
            frame "Jump Train" {
              n344 = Unbundle By Name(w993) -> ("Jump Train"=w992:refnum<vi>)
              n345 = property class="Clust (strict)"(reference=w992, error in=w990) -> (reference out=w991:refnum<vi>, error out=w988:errorcluster, "Value"=w984:T4)
              n346 = call "calc_jumpTrainWaveform_v0.03.vi"("New input cluster"=w984, "Clear Waveform?"=w982, "Old input cluster"=w984, "sample freq"=w985, "Jump Filter Freq (Hz)"=w986, "error in"=w988) -> ("output cluster"=w983:T4, "error out"=w987:errorcluster)  [unwired: 8 in]
              n347 = property class="Clust (strict)"(reference=w991, error in=w987, "Value"=w983) -> (error out=w989:errorcluster)  [unwired: 1 out]
            }
            frame "Voltage Ramp" {
              n348 = Unbundle By Name(w1004) -> ("Voltage Ramp"=w1003:refnum<vi>)
              n349 = property class="Clust (strict)"(reference=w1003, error in=w1001) -> (reference out=w1002:refnum<vi>, error out=w998:errorcluster, "Value"=w996:T5)
              n350 = call "calc_VoltageRampWaveform_v0.03.vi"("New input cluster"=w996, "Clear Waveform?"=w994, "Old input cluster"=w996, "sample freq"=w997, "error in"=w998) -> ("output cluster"=w995:T5, "error out"=w999:errorcluster)  [unwired: 9 in]
              n351 = property class="Clust (strict)"(reference=w1002, error in=w999, "Value"=w995) -> (error out=w1000:errorcluster)  [unwired: 1 out]
            }
            frame "Current Ramp" {
              n352 = Unbundle By Name(w1015) -> ("Current Ramp"=w1014:refnum<vi>)
              n353 = property class="Clust (strict)"(reference=w1014, error in=w1012) -> (reference out=w1013:refnum<vi>, error out=w1009:errorcluster, "Value"=w1007:T6)
              n354 = call "calc_CurrentRampWaveform_v0.03.vi"("New input cluster"=w1007, "Clear Waveform?"=w1005, "Old input cluster"=w1007, "sample freq"=w1008, "error in"=w1009) -> ("output cluster"=w1006:T6, "error out"=w1010:errorcluster)  [unwired: 9 in]
              n355 = property class="Clust (strict)"(reference=w1013, error in=w1010, "Value"=w1006) -> (error out=w1011:errorcluster)  [unwired: 1 out]
            }
            frame "Voltage Step" {
              n356 = Unbundle By Name(w1026) -> ("Voltage Step"=w1025:refnum<vi>)
              n357 = property class="Clust (strict)"(reference=w1025, error in=w1023) -> (reference out=w1024:refnum<vi>, error out=w1020:errorcluster, "Value"=w1018:T7)
              n358 = call "calc_VoltageStepWaveform_v0.03.vi"("New input cluster"=w1018, "Clear Waveform?"=w1016, "Old input cluster"=w1018, "sample freq"=w1019, "error in"=w1020) -> ("output cluster"=w1017:T7, "error out"=w1021:errorcluster)  [unwired: 9 in]
              n359 = property class="Clust (strict)"(reference=w1024, error in=w1021, "Value"=w1017) -> (error out=w1022:errorcluster)  [unwired: 1 out]
            }
            frame "Solution Change" {
              n360 = Unbundle By Name(w1037) -> ("Solution Change"=w1036:refnum<vi>)
              n361 = property class="Clust (strict)"(reference=w1036, error in=w1034) -> (reference out=w1035:refnum<vi>, error out=w1031:errorcluster, "Value"=w1029:T8)
              n362 = call "calc_SolutionChangeWaveform_v0.03.vi"("New input cluster"=w1029, "Clear Waveform?"=w1027, "Old input cluster"=w1029, "sample freq"=w1030, "error in"=w1031) -> ("output cluster"=w1028:T8, "error out"=w1032:errorcluster)  [unwired: 9 in]
              n363 = property class="Clust (strict)"(reference=w1035, error in=w1032, "Value"=w1028) -> (error out=w1033:errorcluster)  [unwired: 1 out]
            }
            frame "Single Jump" {
              n364 = Unbundle By Name(w1049) -> ("Single Jump"=w1048:refnum<vi>)
              n365 = property class="Clust (strict)"(reference=w1048, error in=w1046) -> (reference out=w1047:refnum<vi>, error out=w1044:errorcluster, "Value"=w1041:T9)
              n366 = call "calc_sinlge JumpWaveform_v0.03.vi"("New input cluster"=w1041, "Clear Waveform?"=w1038, "Old input cluster"=w1041, "sample freq"=w1040, "Jump Filter Freq (Hz)"=w1039, "error in"=w1044) -> ("output cluster"=w1042:T9, "error out"=w1043:errorcluster)  [unwired: 8 in]
              n367 = property class="Clust (strict)"(reference=w1047, error in=w1043, "Value"=w1042) -> (error out=w1045:errorcluster)  [unwired: 1 out]
            }
            frame "Single Manip Jump" {
              n368 = Unbundle By Name(w1060) -> ("Single Manip Jump"=w1059:refnum<vi>)
              n369 = property class="Clust (strict)"(reference=w1059, error in=w1057) -> (reference out=w1058:refnum<vi>, error out=w1054:errorcluster, "Value"=w1052:T10)
              n370 = call "calc_singleManipJumpWaveform_v0.02.vi"("New input cluster"=w1052, "Clear Waveform?"=w1050, "Old input cluster"=w1052, "simulate Wave freq"=w1053, "error in"=w1054) -> ("output cluster"=w1051:T10, "error out"=w1055:errorcluster)  [unwired: 9 in]
              n371 = property class="Clust (strict)"(reference=w1058, error in=w1055, "Value"=w1051) -> (error out=w1056:errorcluster)  [unwired: 1 out]
            }
            frame "Multi M. Jump" {
              n372 = Unbundle By Name(w1071) -> ("Multi Manip Jump"=w1070:refnum<vi>)
              n373 = property class="Clust (strict)"(reference=w1070, error in=w1068) -> (reference out=w1069:refnum<vi>, error out=w1065:errorcluster, "Value"=w1063:T11)
              n374 = call "calc_multiManipJumpWaveform_v0.02.vi"("New input cluster"=w1063, "Clear Waveform?"=w1061, "Old input cluster"=w1063, "Numeric"=w1064, "error in"=w1065) -> ("output cluster"=w1062:T11, "error out"=w1066:errorcluster)  [unwired: 9 in]
              n375 = property class="Clust (strict)"(reference=w1069, error in=w1066, "Value"=w1062) -> (error out=w1067:errorcluster)  [unwired: 1 out]
            }
            frame "Voltage Pulse" {
              n376 = Unbundle By Name(w1082) -> ("Voltage Pulse"=w1081:refnum<vi>)
              n377 = property class="Clust (strict)"(reference=w1081, error in=w1079) -> (reference out=w1080:refnum<vi>, error out=w1076:errorcluster, "Value"=w1074:T12)
              n378 = call "calc_VoltagepulseWaveform_v0.03.vi"("New input cluster"=w1074, "Clear Waveform?"=w1072, "Old input cluster"=w1074, "sample freq"=w1075, "error in"=w1076) -> ("output cluster"=w1073:T12, "error out"=w1077:errorcluster)  [unwired: 9 in]
              n379 = property class="Clust (strict)"(reference=w1080, error in=w1077, "Value"=w1073) -> (error out=w1078:errorcluster)  [unwired: 1 out]
            }
            frame "Current Pulse" {
              n380 = Unbundle By Name(w1093) -> ("Current Pulse"=w1092:refnum<vi>)
              n381 = property class="Clust (strict)"(reference=w1092, error in=w1090) -> (reference out=w1091:refnum<vi>, error out=w1087:errorcluster, "Value"=w1085:T13)
              n382 = call "calc_CurrentpulseWaveform_v0.03.vi"("New input cluster"=w1085, "Clear Waveform?"=w1083, "Old input cluster"=w1085, "sample freq"=w1086, "error in"=w1087) -> ("output cluster"=w1084:T13, "error out"=w1088:errorcluster)  [unwired: 9 in]
              n383 = property class="Clust (strict)"(reference=w1091, error in=w1088, "Value"=w1084) -> (error out=w1089:errorcluster)  [unwired: 1 out]
            }
          }
        }
      }
      frame "PhaseH Cluster" {
        # "loop through all exp"
        n384 = Unbundle By Name(w1103) -> ("PhaseA Cluster"=w1102:T2)
        n385 = for {
          tunnel: w1102 -> [w1117]
          tunnel: w1101 -> [w1114] mode=indexing
          tunnel: w1100 -> [w1119]
          tunnel: [w1118] -> w1099
          tunnel: w1098 -> [w1107]
          tunnel: w1097 -> [w1113]
          tunnel: w1096 -> [w1112]
          tunnel: w1095 -> [w1111]
          tunnel: w1094 -> [w1110]
          n386 = Unbundle By Name(w1117) -> ("Phase Experiment Option"=w1116:refnum<vi>)
          n387 = property class="CmbBox"(reference=w1116) -> ("Value"=w1115:string)  [unwired: 1 in, 2 out]
          n388 = Equal?(x=w1115, y=w1114) -> (x = y?=w1108:bool)
          n389 = Greater?(x=w1111, y=w1110) -> (0:w1105:bool)
          n390 = Not(x=w1108) -> (.not. x?=w1109:bool)
          n391 = Select(t=w1107, s=w1107, f=w1109) -> (s? t:f=w1106:bool)
          n392 = Or(x=w1105, y=w1106) -> (x .or. y?=w1104:bool)
          n393 = case shown="\"Current Pulse\"" w1114 {
            tunnel: w1117 -> [w1131 w1143 w1154 w1165 w1176 w1187 w1199 w1210 w1221 w1232 w1243]
            tunnel: w1119 -> [w1127 w1140 w1151 w1162 w1173 w1184 w1196 w1207 w1218 w1229 w1240]
            tunnel: [w1124 w1139 w1150 w1161 w1172 w1183 w1195 w1206 w1217 w1228 w1239] -> w1118
            tunnel: w1113 -> [w1122 w1135 w1147 w1158 w1169 w1180 w1190 w1203 w1214 w1225 w1236]
            tunnel: w1112 -> [w1121 w1136 _ _ _ _ w1189 _ _ _ _]
            tunnel: w1104 -> [w1120 w1132 w1144 w1155 w1166 w1177 w1188 w1200 w1211 w1222 w1233]
            frame "Paired Pulse", Default {
              n394 = Unbundle By Name(w1131) -> ("Paired Pulse"=w1130:refnum<vi>)
              n395 = property class="Clust (strict)"(reference=w1130, error in=w1127) -> (reference out=w1128:refnum<vi>, error out=w1126:errorcluster, "Value"=w1129:T3)
              n396 = call "calc_PairedPulseWaveform_v0.02.vi"("New input cluster"=w1129, "Clear Waveform?"=w1120, "Old input cluster"=w1129, "Numeric"=w1122, "Jump Filter Freq (Hz)"=w1121, "error in"=w1126) -> ("output cluster"=w1123:T3, "error out"=w1125:errorcluster)  [unwired: 8 in]
              n397 = property class="Clust (strict)"(reference=w1128, error in=w1125, "Value"=w1123) -> (error out=w1124:errorcluster)  [unwired: 1 out]
            }
            frame "Jump Train" {
              n398 = Unbundle By Name(w1143) -> ("Jump Train"=w1142:refnum<vi>)
              n399 = property class="Clust (strict)"(reference=w1142, error in=w1140) -> (reference out=w1141:refnum<vi>, error out=w1138:errorcluster, "Value"=w1134:T4)
              n400 = call "calc_jumpTrainWaveform_v0.03.vi"("New input cluster"=w1134, "Clear Waveform?"=w1132, "Old input cluster"=w1134, "sample freq"=w1135, "Jump Filter Freq (Hz)"=w1136, "error in"=w1138) -> ("output cluster"=w1133:T4, "error out"=w1137:errorcluster)  [unwired: 8 in]
              n401 = property class="Clust (strict)"(reference=w1141, error in=w1137, "Value"=w1133) -> (error out=w1139:errorcluster)  [unwired: 1 out]
            }
            frame "Voltage Ramp" {
              n402 = Unbundle By Name(w1154) -> ("Voltage Ramp"=w1153:refnum<vi>)
              n403 = property class="Clust (strict)"(reference=w1153, error in=w1151) -> (reference out=w1152:refnum<vi>, error out=w1148:errorcluster, "Value"=w1146:T5)
              n404 = call "calc_VoltageRampWaveform_v0.03.vi"("New input cluster"=w1146, "Clear Waveform?"=w1144, "Old input cluster"=w1146, "sample freq"=w1147, "error in"=w1148) -> ("output cluster"=w1145:T5, "error out"=w1149:errorcluster)  [unwired: 9 in]
              n405 = property class="Clust (strict)"(reference=w1152, error in=w1149, "Value"=w1145) -> (error out=w1150:errorcluster)  [unwired: 1 out]
            }
            frame "Current Ramp" {
              n406 = Unbundle By Name(w1165) -> ("Current Ramp"=w1164:refnum<vi>)
              n407 = property class="Clust (strict)"(reference=w1164, error in=w1162) -> (reference out=w1163:refnum<vi>, error out=w1159:errorcluster, "Value"=w1157:T6)
              n408 = call "calc_CurrentRampWaveform_v0.03.vi"("New input cluster"=w1157, "Clear Waveform?"=w1155, "Old input cluster"=w1157, "sample freq"=w1158, "error in"=w1159) -> ("output cluster"=w1156:T6, "error out"=w1160:errorcluster)  [unwired: 9 in]
              n409 = property class="Clust (strict)"(reference=w1163, error in=w1160, "Value"=w1156) -> (error out=w1161:errorcluster)  [unwired: 1 out]
            }
            frame "Voltage Step" {
              n410 = Unbundle By Name(w1176) -> ("Voltage Step"=w1175:refnum<vi>)
              n411 = property class="Clust (strict)"(reference=w1175, error in=w1173) -> (reference out=w1174:refnum<vi>, error out=w1170:errorcluster, "Value"=w1168:T7)
              n412 = call "calc_VoltageStepWaveform_v0.03.vi"("New input cluster"=w1168, "Clear Waveform?"=w1166, "Old input cluster"=w1168, "sample freq"=w1169, "error in"=w1170) -> ("output cluster"=w1167:T7, "error out"=w1171:errorcluster)  [unwired: 9 in]
              n413 = property class="Clust (strict)"(reference=w1174, error in=w1171, "Value"=w1167) -> (error out=w1172:errorcluster)  [unwired: 1 out]
            }
            frame "Solution Change" {
              n414 = Unbundle By Name(w1187) -> ("Solution Change"=w1186:refnum<vi>)
              n415 = property class="Clust (strict)"(reference=w1186, error in=w1184) -> (reference out=w1185:refnum<vi>, error out=w1181:errorcluster, "Value"=w1179:T8)
              n416 = call "calc_SolutionChangeWaveform_v0.03.vi"("New input cluster"=w1179, "Clear Waveform?"=w1177, "Old input cluster"=w1179, "sample freq"=w1180, "error in"=w1181) -> ("output cluster"=w1178:T8, "error out"=w1182:errorcluster)  [unwired: 9 in]
              n417 = property class="Clust (strict)"(reference=w1185, error in=w1182, "Value"=w1178) -> (error out=w1183:errorcluster)  [unwired: 1 out]
            }
            frame "Single Jump" {
              n418 = Unbundle By Name(w1199) -> ("Single Jump"=w1198:refnum<vi>)
              n419 = property class="Clust (strict)"(reference=w1198, error in=w1196) -> (reference out=w1197:refnum<vi>, error out=w1194:errorcluster, "Value"=w1191:T9)
              n420 = call "calc_sinlge JumpWaveform_v0.03.vi"("New input cluster"=w1191, "Clear Waveform?"=w1188, "Old input cluster"=w1191, "sample freq"=w1190, "Jump Filter Freq (Hz)"=w1189, "error in"=w1194) -> ("output cluster"=w1192:T9, "error out"=w1193:errorcluster)  [unwired: 8 in]
              n421 = property class="Clust (strict)"(reference=w1197, error in=w1193, "Value"=w1192) -> (error out=w1195:errorcluster)  [unwired: 1 out]
            }
            frame "Single Manip Jump" {
              n422 = Unbundle By Name(w1210) -> ("Single Manip Jump"=w1209:refnum<vi>)
              n423 = property class="Clust (strict)"(reference=w1209, error in=w1207) -> (reference out=w1208:refnum<vi>, error out=w1204:errorcluster, "Value"=w1202:T10)
              n424 = call "calc_singleManipJumpWaveform_v0.02.vi"("New input cluster"=w1202, "Clear Waveform?"=w1200, "Old input cluster"=w1202, "simulate Wave freq"=w1203, "error in"=w1204) -> ("output cluster"=w1201:T10, "error out"=w1205:errorcluster)  [unwired: 9 in]
              n425 = property class="Clust (strict)"(reference=w1208, error in=w1205, "Value"=w1201) -> (error out=w1206:errorcluster)  [unwired: 1 out]
            }
            frame "Multi M. Jump" {
              n426 = Unbundle By Name(w1221) -> ("Multi Manip Jump"=w1220:refnum<vi>)
              n427 = property class="Clust (strict)"(reference=w1220, error in=w1218) -> (reference out=w1219:refnum<vi>, error out=w1215:errorcluster, "Value"=w1213:T11)
              n428 = call "calc_multiManipJumpWaveform_v0.02.vi"("New input cluster"=w1213, "Clear Waveform?"=w1211, "Old input cluster"=w1213, "Numeric"=w1214, "error in"=w1215) -> ("output cluster"=w1212:T11, "error out"=w1216:errorcluster)  [unwired: 9 in]
              n429 = property class="Clust (strict)"(reference=w1219, error in=w1216, "Value"=w1212) -> (error out=w1217:errorcluster)  [unwired: 1 out]
            }
            frame "Voltage Pulse" {
              n430 = Unbundle By Name(w1232) -> ("Voltage Pulse"=w1231:refnum<vi>)
              n431 = property class="Clust (strict)"(reference=w1231, error in=w1229) -> (reference out=w1230:refnum<vi>, error out=w1226:errorcluster, "Value"=w1224:T12)
              n432 = call "calc_VoltagepulseWaveform_v0.03.vi"("New input cluster"=w1224, "Clear Waveform?"=w1222, "Old input cluster"=w1224, "sample freq"=w1225, "error in"=w1226) -> ("output cluster"=w1223:T12, "error out"=w1227:errorcluster)  [unwired: 9 in]
              n433 = property class="Clust (strict)"(reference=w1230, error in=w1227, "Value"=w1223) -> (error out=w1228:errorcluster)  [unwired: 1 out]
            }
            frame "Current Pulse" {
              n434 = Unbundle By Name(w1243) -> ("Current Pulse"=w1242:refnum<vi>)
              n435 = property class="Clust (strict)"(reference=w1242, error in=w1240) -> (reference out=w1241:refnum<vi>, error out=w1237:errorcluster, "Value"=w1235:T13)
              n436 = call "calc_CurrentpulseWaveform_v0.03.vi"("New input cluster"=w1235, "Clear Waveform?"=w1233, "Old input cluster"=w1235, "sample freq"=w1236, "error in"=w1237) -> ("output cluster"=w1234:T13, "error out"=w1238:errorcluster)  [unwired: 9 in]
              n437 = property class="Clust (strict)"(reference=w1241, error in=w1238, "Value"=w1234) -> (error out=w1239:errorcluster)  [unwired: 1 out]
            }
          }
        }
      }
      frame "PhaseI Cluster" {
        # "loop through all exp"
        n438 = Unbundle By Name(w1253) -> ("PhaseA Cluster"=w1252:T2)
        n439 = for {
          tunnel: w1252 -> [w1267]
          tunnel: w1251 -> [w1264] mode=indexing
          tunnel: w1250 -> [w1269]
          tunnel: [w1268] -> w1249
          tunnel: w1248 -> [w1257]
          tunnel: w1247 -> [w1263]
          tunnel: w1246 -> [w1262]
          tunnel: w1245 -> [w1261]
          tunnel: w1244 -> [w1260]
          n440 = Unbundle By Name(w1267) -> ("Phase Experiment Option"=w1266:refnum<vi>)
          n441 = property class="CmbBox"(reference=w1266) -> ("Value"=w1265:string)  [unwired: 1 in, 2 out]
          n442 = Equal?(x=w1265, y=w1264) -> (x = y?=w1258:bool)
          n443 = Greater?(x=w1261, y=w1260) -> (0:w1255:bool)
          n444 = Not(x=w1258) -> (.not. x?=w1259:bool)
          n445 = Select(t=w1257, s=w1257, f=w1259) -> (s? t:f=w1256:bool)
          n446 = Or(x=w1255, y=w1256) -> (x .or. y?=w1254:bool)
          n447 = case shown="\"Current Pulse\"" w1264 {
            tunnel: w1267 -> [w1281 w1293 w1304 w1315 w1326 w1337 w1349 w1360 w1371 w1382 w1393]
            tunnel: w1269 -> [w1277 w1290 w1301 w1312 w1323 w1334 w1346 w1357 w1368 w1379 w1390]
            tunnel: [w1274 w1289 w1300 w1311 w1322 w1333 w1345 w1356 w1367 w1378 w1389] -> w1268
            tunnel: w1263 -> [w1272 w1285 w1297 w1308 w1319 w1330 w1340 w1353 w1364 w1375 w1386]
            tunnel: w1262 -> [w1271 w1286 _ _ _ _ w1339 _ _ _ _]
            tunnel: w1254 -> [w1270 w1282 w1294 w1305 w1316 w1327 w1338 w1350 w1361 w1372 w1383]
            frame "Paired Pulse", Default {
              n448 = Unbundle By Name(w1281) -> ("Paired Pulse"=w1280:refnum<vi>)
              n449 = property class="Clust (strict)"(reference=w1280, error in=w1277) -> (reference out=w1278:refnum<vi>, error out=w1276:errorcluster, "Value"=w1279:T3)
              n450 = call "calc_PairedPulseWaveform_v0.02.vi"("New input cluster"=w1279, "Clear Waveform?"=w1270, "Old input cluster"=w1279, "Numeric"=w1272, "Jump Filter Freq (Hz)"=w1271, "error in"=w1276) -> ("output cluster"=w1273:T3, "error out"=w1275:errorcluster)  [unwired: 8 in]
              n451 = property class="Clust (strict)"(reference=w1278, error in=w1275, "Value"=w1273) -> (error out=w1274:errorcluster)  [unwired: 1 out]
            }
            frame "Jump Train" {
              n452 = Unbundle By Name(w1293) -> ("Jump Train"=w1292:refnum<vi>)
              n453 = property class="Clust (strict)"(reference=w1292, error in=w1290) -> (reference out=w1291:refnum<vi>, error out=w1288:errorcluster, "Value"=w1284:T4)
              n454 = call "calc_jumpTrainWaveform_v0.03.vi"("New input cluster"=w1284, "Clear Waveform?"=w1282, "Old input cluster"=w1284, "sample freq"=w1285, "Jump Filter Freq (Hz)"=w1286, "error in"=w1288) -> ("output cluster"=w1283:T4, "error out"=w1287:errorcluster)  [unwired: 8 in]
              n455 = property class="Clust (strict)"(reference=w1291, error in=w1287, "Value"=w1283) -> (error out=w1289:errorcluster)  [unwired: 1 out]
            }
            frame "Voltage Ramp" {
              n456 = Unbundle By Name(w1304) -> ("Voltage Ramp"=w1303:refnum<vi>)
              n457 = property class="Clust (strict)"(reference=w1303, error in=w1301) -> (reference out=w1302:refnum<vi>, error out=w1298:errorcluster, "Value"=w1296:T5)
              n458 = call "calc_VoltageRampWaveform_v0.03.vi"("New input cluster"=w1296, "Clear Waveform?"=w1294, "Old input cluster"=w1296, "sample freq"=w1297, "error in"=w1298) -> ("output cluster"=w1295:T5, "error out"=w1299:errorcluster)  [unwired: 9 in]
              n459 = property class="Clust (strict)"(reference=w1302, error in=w1299, "Value"=w1295) -> (error out=w1300:errorcluster)  [unwired: 1 out]
            }
            frame "Current Ramp" {
              n460 = Unbundle By Name(w1315) -> ("Current Ramp"=w1314:refnum<vi>)
              n461 = property class="Clust (strict)"(reference=w1314, error in=w1312) -> (reference out=w1313:refnum<vi>, error out=w1309:errorcluster, "Value"=w1307:T6)
              n462 = call "calc_CurrentRampWaveform_v0.03.vi"("New input cluster"=w1307, "Clear Waveform?"=w1305, "Old input cluster"=w1307, "sample freq"=w1308, "error in"=w1309) -> ("output cluster"=w1306:T6, "error out"=w1310:errorcluster)  [unwired: 9 in]
              n463 = property class="Clust (strict)"(reference=w1313, error in=w1310, "Value"=w1306) -> (error out=w1311:errorcluster)  [unwired: 1 out]
            }
            frame "Voltage Step" {
              n464 = Unbundle By Name(w1326) -> ("Voltage Step"=w1325:refnum<vi>)
              n465 = property class="Clust (strict)"(reference=w1325, error in=w1323) -> (reference out=w1324:refnum<vi>, error out=w1320:errorcluster, "Value"=w1318:T7)
              n466 = call "calc_VoltageStepWaveform_v0.03.vi"("New input cluster"=w1318, "Clear Waveform?"=w1316, "Old input cluster"=w1318, "sample freq"=w1319, "error in"=w1320) -> ("output cluster"=w1317:T7, "error out"=w1321:errorcluster)  [unwired: 9 in]
              n467 = property class="Clust (strict)"(reference=w1324, error in=w1321, "Value"=w1317) -> (error out=w1322:errorcluster)  [unwired: 1 out]
            }
            frame "Solution Change" {
              n468 = Unbundle By Name(w1337) -> ("Solution Change"=w1336:refnum<vi>)
              n469 = property class="Clust (strict)"(reference=w1336, error in=w1334) -> (reference out=w1335:refnum<vi>, error out=w1331:errorcluster, "Value"=w1329:T8)
              n470 = call "calc_SolutionChangeWaveform_v0.03.vi"("New input cluster"=w1329, "Clear Waveform?"=w1327, "Old input cluster"=w1329, "sample freq"=w1330, "error in"=w1331) -> ("output cluster"=w1328:T8, "error out"=w1332:errorcluster)  [unwired: 9 in]
              n471 = property class="Clust (strict)"(reference=w1335, error in=w1332, "Value"=w1328) -> (error out=w1333:errorcluster)  [unwired: 1 out]
            }
            frame "Single Jump" {
              n472 = Unbundle By Name(w1349) -> ("Single Jump"=w1348:refnum<vi>)
              n473 = property class="Clust (strict)"(reference=w1348, error in=w1346) -> (reference out=w1347:refnum<vi>, error out=w1344:errorcluster, "Value"=w1341:T9)
              n474 = call "calc_sinlge JumpWaveform_v0.03.vi"("New input cluster"=w1341, "Clear Waveform?"=w1338, "Old input cluster"=w1341, "sample freq"=w1340, "Jump Filter Freq (Hz)"=w1339, "error in"=w1344) -> ("output cluster"=w1342:T9, "error out"=w1343:errorcluster)  [unwired: 8 in]
              n475 = property class="Clust (strict)"(reference=w1347, error in=w1343, "Value"=w1342) -> (error out=w1345:errorcluster)  [unwired: 1 out]
            }
            frame "Single Manip Jump" {
              n476 = Unbundle By Name(w1360) -> ("Single Manip Jump"=w1359:refnum<vi>)
              n477 = property class="Clust (strict)"(reference=w1359, error in=w1357) -> (reference out=w1358:refnum<vi>, error out=w1354:errorcluster, "Value"=w1352:T10)
              n478 = call "calc_singleManipJumpWaveform_v0.02.vi"("New input cluster"=w1352, "Clear Waveform?"=w1350, "Old input cluster"=w1352, "simulate Wave freq"=w1353, "error in"=w1354) -> ("output cluster"=w1351:T10, "error out"=w1355:errorcluster)  [unwired: 9 in]
              n479 = property class="Clust (strict)"(reference=w1358, error in=w1355, "Value"=w1351) -> (error out=w1356:errorcluster)  [unwired: 1 out]
            }
            frame "Multi M. Jump" {
              n480 = Unbundle By Name(w1371) -> ("Multi Manip Jump"=w1370:refnum<vi>)
              n481 = property class="Clust (strict)"(reference=w1370, error in=w1368) -> (reference out=w1369:refnum<vi>, error out=w1365:errorcluster, "Value"=w1363:T11)
              n482 = call "calc_multiManipJumpWaveform_v0.02.vi"("New input cluster"=w1363, "Clear Waveform?"=w1361, "Old input cluster"=w1363, "Numeric"=w1364, "error in"=w1365) -> ("output cluster"=w1362:T11, "error out"=w1366:errorcluster)  [unwired: 9 in]
              n483 = property class="Clust (strict)"(reference=w1369, error in=w1366, "Value"=w1362) -> (error out=w1367:errorcluster)  [unwired: 1 out]
            }
            frame "Voltage Pulse" {
              n484 = Unbundle By Name(w1382) -> ("Voltage Pulse"=w1381:refnum<vi>)
              n485 = property class="Clust (strict)"(reference=w1381, error in=w1379) -> (reference out=w1380:refnum<vi>, error out=w1376:errorcluster, "Value"=w1374:T12)
              n486 = call "calc_VoltagepulseWaveform_v0.03.vi"("New input cluster"=w1374, "Clear Waveform?"=w1372, "Old input cluster"=w1374, "sample freq"=w1375, "error in"=w1376) -> ("output cluster"=w1373:T12, "error out"=w1377:errorcluster)  [unwired: 9 in]
              n487 = property class="Clust (strict)"(reference=w1380, error in=w1377, "Value"=w1373) -> (error out=w1378:errorcluster)  [unwired: 1 out]
            }
            frame "Current Pulse" {
              n488 = Unbundle By Name(w1393) -> ("Current Pulse"=w1392:refnum<vi>)
              n489 = property class="Clust (strict)"(reference=w1392, error in=w1390) -> (reference out=w1391:refnum<vi>, error out=w1387:errorcluster, "Value"=w1385:T13)
              n490 = call "calc_CurrentpulseWaveform_v0.03.vi"("New input cluster"=w1385, "Clear Waveform?"=w1383, "Old input cluster"=w1385, "sample freq"=w1386, "error in"=w1387) -> ("output cluster"=w1384:T13, "error out"=w1388:errorcluster)  [unwired: 9 in]
              n491 = property class="Clust (strict)"(reference=w1391, error in=w1388, "Value"=w1384) -> (error out=w1389:errorcluster)  [unwired: 1 out]
            }
          }
        }
      }
      frame "PhaseJ Cluster" {
        # "loop through all exp"
        n492 = Unbundle By Name(w1403) -> ("PhaseA Cluster"=w1402:T2)
        n493 = for {
          tunnel: w1402 -> [w1417]
          tunnel: w1401 -> [w1414] mode=indexing
          tunnel: w1400 -> [w1419]
          tunnel: [w1418] -> w1399
          tunnel: w1398 -> [w1407]
          tunnel: w1397 -> [w1413]
          tunnel: w1396 -> [w1412]
          tunnel: w1395 -> [w1411]
          tunnel: w1394 -> [w1410]
          n494 = Unbundle By Name(w1417) -> ("Phase Experiment Option"=w1416:refnum<vi>)
          n495 = property class="CmbBox"(reference=w1416) -> ("Value"=w1415:string)  [unwired: 1 in, 2 out]
          n496 = Equal?(x=w1415, y=w1414) -> (x = y?=w1408:bool)
          n497 = Greater?(x=w1411, y=w1410) -> (0:w1405:bool)
          n498 = Not(x=w1408) -> (.not. x?=w1409:bool)
          n499 = Select(t=w1407, s=w1407, f=w1409) -> (s? t:f=w1406:bool)
          n500 = Or(x=w1405, y=w1406) -> (x .or. y?=w1404:bool)
          n501 = case shown="\"Current Pulse\"" w1414 {
            tunnel: w1417 -> [w1431 w1443 w1454 w1465 w1476 w1487 w1499 w1510 w1521 w1532 w1543]
            tunnel: w1419 -> [w1427 w1440 w1451 w1462 w1473 w1484 w1496 w1507 w1518 w1529 w1540]
            tunnel: [w1424 w1439 w1450 w1461 w1472 w1483 w1495 w1506 w1517 w1528 w1539] -> w1418
            tunnel: w1413 -> [w1422 w1435 w1447 w1458 w1469 w1480 w1490 w1503 w1514 w1525 w1536]
            tunnel: w1412 -> [w1421 w1436 _ _ _ _ w1489 _ _ _ _]
            tunnel: w1404 -> [w1420 w1432 w1444 w1455 w1466 w1477 w1488 w1500 w1511 w1522 w1533]
            frame "Paired Pulse", Default {
              n502 = Unbundle By Name(w1431) -> ("Paired Pulse"=w1430:refnum<vi>)
              n503 = property class="Clust (strict)"(reference=w1430, error in=w1427) -> (reference out=w1428:refnum<vi>, error out=w1426:errorcluster, "Value"=w1429:T3)
              n504 = call "calc_PairedPulseWaveform_v0.02.vi"("New input cluster"=w1429, "Clear Waveform?"=w1420, "Old input cluster"=w1429, "Numeric"=w1422, "Jump Filter Freq (Hz)"=w1421, "error in"=w1426) -> ("output cluster"=w1423:T3, "error out"=w1425:errorcluster)  [unwired: 8 in]
              n505 = property class="Clust (strict)"(reference=w1428, error in=w1425, "Value"=w1423) -> (error out=w1424:errorcluster)  [unwired: 1 out]
            }
            frame "Jump Train" {
              n506 = Unbundle By Name(w1443) -> ("Jump Train"=w1442:refnum<vi>)
              n507 = property class="Clust (strict)"(reference=w1442, error in=w1440) -> (reference out=w1441:refnum<vi>, error out=w1438:errorcluster, "Value"=w1434:T4)
              n508 = call "calc_jumpTrainWaveform_v0.03.vi"("New input cluster"=w1434, "Clear Waveform?"=w1432, "Old input cluster"=w1434, "sample freq"=w1435, "Jump Filter Freq (Hz)"=w1436, "error in"=w1438) -> ("output cluster"=w1433:T4, "error out"=w1437:errorcluster)  [unwired: 8 in]
              n509 = property class="Clust (strict)"(reference=w1441, error in=w1437, "Value"=w1433) -> (error out=w1439:errorcluster)  [unwired: 1 out]
            }
            frame "Voltage Ramp" {
              n510 = Unbundle By Name(w1454) -> ("Voltage Ramp"=w1453:refnum<vi>)
              n511 = property class="Clust (strict)"(reference=w1453, error in=w1451) -> (reference out=w1452:refnum<vi>, error out=w1448:errorcluster, "Value"=w1446:T5)
              n512 = call "calc_VoltageRampWaveform_v0.03.vi"("New input cluster"=w1446, "Clear Waveform?"=w1444, "Old input cluster"=w1446, "sample freq"=w1447, "error in"=w1448) -> ("output cluster"=w1445:T5, "error out"=w1449:errorcluster)  [unwired: 9 in]
              n513 = property class="Clust (strict)"(reference=w1452, error in=w1449, "Value"=w1445) -> (error out=w1450:errorcluster)  [unwired: 1 out]
            }
            frame "Current Ramp" {
              n514 = Unbundle By Name(w1465) -> ("Current Ramp"=w1464:refnum<vi>)
              n515 = property class="Clust (strict)"(reference=w1464, error in=w1462) -> (reference out=w1463:refnum<vi>, error out=w1459:errorcluster, "Value"=w1457:T6)
              n516 = call "calc_CurrentRampWaveform_v0.03.vi"("New input cluster"=w1457, "Clear Waveform?"=w1455, "Old input cluster"=w1457, "sample freq"=w1458, "error in"=w1459) -> ("output cluster"=w1456:T6, "error out"=w1460:errorcluster)  [unwired: 9 in]
              n517 = property class="Clust (strict)"(reference=w1463, error in=w1460, "Value"=w1456) -> (error out=w1461:errorcluster)  [unwired: 1 out]
            }
            frame "Voltage Step" {
              n518 = Unbundle By Name(w1476) -> ("Voltage Step"=w1475:refnum<vi>)
              n519 = property class="Clust (strict)"(reference=w1475, error in=w1473) -> (reference out=w1474:refnum<vi>, error out=w1470:errorcluster, "Value"=w1468:T7)
              n520 = call "calc_VoltageStepWaveform_v0.03.vi"("New input cluster"=w1468, "Clear Waveform?"=w1466, "Old input cluster"=w1468, "sample freq"=w1469, "error in"=w1470) -> ("output cluster"=w1467:T7, "error out"=w1471:errorcluster)  [unwired: 9 in]
              n521 = property class="Clust (strict)"(reference=w1474, error in=w1471, "Value"=w1467) -> (error out=w1472:errorcluster)  [unwired: 1 out]
            }
            frame "Solution Change" {
              n522 = Unbundle By Name(w1487) -> ("Solution Change"=w1486:refnum<vi>)
              n523 = property class="Clust (strict)"(reference=w1486, error in=w1484) -> (reference out=w1485:refnum<vi>, error out=w1481:errorcluster, "Value"=w1479:T8)
              n524 = call "calc_SolutionChangeWaveform_v0.03.vi"("New input cluster"=w1479, "Clear Waveform?"=w1477, "Old input cluster"=w1479, "sample freq"=w1480, "error in"=w1481) -> ("output cluster"=w1478:T8, "error out"=w1482:errorcluster)  [unwired: 9 in]
              n525 = property class="Clust (strict)"(reference=w1485, error in=w1482, "Value"=w1478) -> (error out=w1483:errorcluster)  [unwired: 1 out]
            }
            frame "Single Jump" {
              n526 = Unbundle By Name(w1499) -> ("Single Jump"=w1498:refnum<vi>)
              n527 = property class="Clust (strict)"(reference=w1498, error in=w1496) -> (reference out=w1497:refnum<vi>, error out=w1494:errorcluster, "Value"=w1491:T9)
              n528 = call "calc_sinlge JumpWaveform_v0.03.vi"("New input cluster"=w1491, "Clear Waveform?"=w1488, "Old input cluster"=w1491, "sample freq"=w1490, "Jump Filter Freq (Hz)"=w1489, "error in"=w1494) -> ("output cluster"=w1492:T9, "error out"=w1493:errorcluster)  [unwired: 8 in]
              n529 = property class="Clust (strict)"(reference=w1497, error in=w1493, "Value"=w1492) -> (error out=w1495:errorcluster)  [unwired: 1 out]
            }
            frame "Single Manip Jump" {
              n530 = Unbundle By Name(w1510) -> ("Single Manip Jump"=w1509:refnum<vi>)
              n531 = property class="Clust (strict)"(reference=w1509, error in=w1507) -> (reference out=w1508:refnum<vi>, error out=w1504:errorcluster, "Value"=w1502:T10)
              n532 = call "calc_singleManipJumpWaveform_v0.02.vi"("New input cluster"=w1502, "Clear Waveform?"=w1500, "Old input cluster"=w1502, "simulate Wave freq"=w1503, "error in"=w1504) -> ("output cluster"=w1501:T10, "error out"=w1505:errorcluster)  [unwired: 9 in]
              n533 = property class="Clust (strict)"(reference=w1508, error in=w1505, "Value"=w1501) -> (error out=w1506:errorcluster)  [unwired: 1 out]
            }
            frame "Multi M. Jump" {
              n534 = Unbundle By Name(w1521) -> ("Multi Manip Jump"=w1520:refnum<vi>)
              n535 = property class="Clust (strict)"(reference=w1520, error in=w1518) -> (reference out=w1519:refnum<vi>, error out=w1515:errorcluster, "Value"=w1513:T11)
              n536 = call "calc_multiManipJumpWaveform_v0.02.vi"("New input cluster"=w1513, "Clear Waveform?"=w1511, "Old input cluster"=w1513, "Numeric"=w1514, "error in"=w1515) -> ("output cluster"=w1512:T11, "error out"=w1516:errorcluster)  [unwired: 9 in]
              n537 = property class="Clust (strict)"(reference=w1519, error in=w1516, "Value"=w1512) -> (error out=w1517:errorcluster)  [unwired: 1 out]
            }
            frame "Voltage Pulse" {
              n538 = Unbundle By Name(w1532) -> ("Voltage Pulse"=w1531:refnum<vi>)
              n539 = property class="Clust (strict)"(reference=w1531, error in=w1529) -> (reference out=w1530:refnum<vi>, error out=w1526:errorcluster, "Value"=w1524:T12)
              n540 = call "calc_VoltagepulseWaveform_v0.03.vi"("New input cluster"=w1524, "Clear Waveform?"=w1522, "Old input cluster"=w1524, "sample freq"=w1525, "error in"=w1526) -> ("output cluster"=w1523:T12, "error out"=w1527:errorcluster)  [unwired: 9 in]
              n541 = property class="Clust (strict)"(reference=w1530, error in=w1527, "Value"=w1523) -> (error out=w1528:errorcluster)  [unwired: 1 out]
            }
            frame "Current Pulse" {
              n542 = Unbundle By Name(w1543) -> ("Current Pulse"=w1542:refnum<vi>)
              n543 = property class="Clust (strict)"(reference=w1542, error in=w1540) -> (reference out=w1541:refnum<vi>, error out=w1537:errorcluster, "Value"=w1535:T13)
              n544 = call "calc_CurrentpulseWaveform_v0.03.vi"("New input cluster"=w1535, "Clear Waveform?"=w1533, "Old input cluster"=w1535, "sample freq"=w1536, "error in"=w1537) -> ("output cluster"=w1534:T13, "error out"=w1538:errorcluster)  [unwired: 9 in]
              n545 = property class="Clust (strict)"(reference=w1541, error in=w1538, "Value"=w1534) -> (error out=w1539:errorcluster)  [unwired: 1 out]
            }
          }
        }
      }
      frame "PhaseK Cluster" {
        # "loop through all exp"
        n546 = Unbundle By Name(w1553) -> ("PhaseA Cluster"=w1552:T2)
        n547 = for {
          tunnel: w1552 -> [w1567]
          tunnel: w1551 -> [w1564] mode=indexing
          tunnel: w1550 -> [w1569]
          tunnel: [w1568] -> w1549
          tunnel: w1548 -> [w1557]
          tunnel: w1547 -> [w1563]
          tunnel: w1546 -> [w1562]
          tunnel: w1545 -> [w1561]
          tunnel: w1544 -> [w1560]
          n548 = Unbundle By Name(w1567) -> ("Phase Experiment Option"=w1566:refnum<vi>)
          n549 = property class="CmbBox"(reference=w1566) -> ("Value"=w1565:string)  [unwired: 1 in, 2 out]
          n550 = Equal?(x=w1565, y=w1564) -> (x = y?=w1558:bool)
          n551 = Greater?(x=w1561, y=w1560) -> (0:w1555:bool)
          n552 = Not(x=w1558) -> (.not. x?=w1559:bool)
          n553 = Select(t=w1557, s=w1557, f=w1559) -> (s? t:f=w1556:bool)
          n554 = Or(x=w1555, y=w1556) -> (x .or. y?=w1554:bool)
          n555 = case shown="\"Current Pulse\"" w1564 {
            tunnel: w1567 -> [w1581 w1593 w1604 w1615 w1626 w1637 w1649 w1660 w1671 w1682 w1693]
            tunnel: w1569 -> [w1577 w1590 w1601 w1612 w1623 w1634 w1646 w1657 w1668 w1679 w1690]
            tunnel: [w1574 w1589 w1600 w1611 w1622 w1633 w1645 w1656 w1667 w1678 w1689] -> w1568
            tunnel: w1563 -> [w1572 w1585 w1597 w1608 w1619 w1630 w1640 w1653 w1664 w1675 w1686]
            tunnel: w1562 -> [w1571 w1586 _ _ _ _ w1639 _ _ _ _]
            tunnel: w1554 -> [w1570 w1582 w1594 w1605 w1616 w1627 w1638 w1650 w1661 w1672 w1683]
            frame "Paired Pulse", Default {
              n556 = Unbundle By Name(w1581) -> ("Paired Pulse"=w1580:refnum<vi>)
              n557 = property class="Clust (strict)"(reference=w1580, error in=w1577) -> (reference out=w1578:refnum<vi>, error out=w1576:errorcluster, "Value"=w1579:T3)
              n558 = call "calc_PairedPulseWaveform_v0.02.vi"("New input cluster"=w1579, "Clear Waveform?"=w1570, "Old input cluster"=w1579, "Numeric"=w1572, "Jump Filter Freq (Hz)"=w1571, "error in"=w1576) -> ("output cluster"=w1573:T3, "error out"=w1575:errorcluster)  [unwired: 8 in]
              n559 = property class="Clust (strict)"(reference=w1578, error in=w1575, "Value"=w1573) -> (error out=w1574:errorcluster)  [unwired: 1 out]
            }
            frame "Jump Train" {
              n560 = Unbundle By Name(w1593) -> ("Jump Train"=w1592:refnum<vi>)
              n561 = property class="Clust (strict)"(reference=w1592, error in=w1590) -> (reference out=w1591:refnum<vi>, error out=w1588:errorcluster, "Value"=w1584:T4)
              n562 = call "calc_jumpTrainWaveform_v0.03.vi"("New input cluster"=w1584, "Clear Waveform?"=w1582, "Old input cluster"=w1584, "sample freq"=w1585, "Jump Filter Freq (Hz)"=w1586, "error in"=w1588) -> ("output cluster"=w1583:T4, "error out"=w1587:errorcluster)  [unwired: 8 in]
              n563 = property class="Clust (strict)"(reference=w1591, error in=w1587, "Value"=w1583) -> (error out=w1589:errorcluster)  [unwired: 1 out]
            }
            frame "Voltage Ramp" {
              n564 = Unbundle By Name(w1604) -> ("Voltage Ramp"=w1603:refnum<vi>)
              n565 = property class="Clust (strict)"(reference=w1603, error in=w1601) -> (reference out=w1602:refnum<vi>, error out=w1598:errorcluster, "Value"=w1596:T5)
              n566 = call "calc_VoltageRampWaveform_v0.03.vi"("New input cluster"=w1596, "Clear Waveform?"=w1594, "Old input cluster"=w1596, "sample freq"=w1597, "error in"=w1598) -> ("output cluster"=w1595:T5, "error out"=w1599:errorcluster)  [unwired: 9 in]
              n567 = property class="Clust (strict)"(reference=w1602, error in=w1599, "Value"=w1595) -> (error out=w1600:errorcluster)  [unwired: 1 out]
            }
            frame "Current Ramp" {
              n568 = Unbundle By Name(w1615) -> ("Current Ramp"=w1614:refnum<vi>)
              n569 = property class="Clust (strict)"(reference=w1614, error in=w1612) -> (reference out=w1613:refnum<vi>, error out=w1609:errorcluster, "Value"=w1607:T6)
              n570 = call "calc_CurrentRampWaveform_v0.03.vi"("New input cluster"=w1607, "Clear Waveform?"=w1605, "Old input cluster"=w1607, "sample freq"=w1608, "error in"=w1609) -> ("output cluster"=w1606:T6, "error out"=w1610:errorcluster)  [unwired: 9 in]
              n571 = property class="Clust (strict)"(reference=w1613, error in=w1610, "Value"=w1606) -> (error out=w1611:errorcluster)  [unwired: 1 out]
            }
            frame "Voltage Step" {
              n572 = Unbundle By Name(w1626) -> ("Voltage Step"=w1625:refnum<vi>)
              n573 = property class="Clust (strict)"(reference=w1625, error in=w1623) -> (reference out=w1624:refnum<vi>, error out=w1620:errorcluster, "Value"=w1618:T7)
              n574 = call "calc_VoltageStepWaveform_v0.03.vi"("New input cluster"=w1618, "Clear Waveform?"=w1616, "Old input cluster"=w1618, "sample freq"=w1619, "error in"=w1620) -> ("output cluster"=w1617:T7, "error out"=w1621:errorcluster)  [unwired: 9 in]
              n575 = property class="Clust (strict)"(reference=w1624, error in=w1621, "Value"=w1617) -> (error out=w1622:errorcluster)  [unwired: 1 out]
            }
            frame "Solution Change" {
              n576 = Unbundle By Name(w1637) -> ("Solution Change"=w1636:refnum<vi>)
              n577 = property class="Clust (strict)"(reference=w1636, error in=w1634) -> (reference out=w1635:refnum<vi>, error out=w1631:errorcluster, "Value"=w1629:T8)
              n578 = call "calc_SolutionChangeWaveform_v0.03.vi"("New input cluster"=w1629, "Clear Waveform?"=w1627, "Old input cluster"=w1629, "sample freq"=w1630, "error in"=w1631) -> ("output cluster"=w1628:T8, "error out"=w1632:errorcluster)  [unwired: 9 in]
              n579 = property class="Clust (strict)"(reference=w1635, error in=w1632, "Value"=w1628) -> (error out=w1633:errorcluster)  [unwired: 1 out]
            }
            frame "Single Jump" {
              n580 = Unbundle By Name(w1649) -> ("Single Jump"=w1648:refnum<vi>)
              n581 = property class="Clust (strict)"(reference=w1648, error in=w1646) -> (reference out=w1647:refnum<vi>, error out=w1644:errorcluster, "Value"=w1641:T9)
              n582 = call "calc_sinlge JumpWaveform_v0.03.vi"("New input cluster"=w1641, "Clear Waveform?"=w1638, "Old input cluster"=w1641, "sample freq"=w1640, "Jump Filter Freq (Hz)"=w1639, "error in"=w1644) -> ("output cluster"=w1642:T9, "error out"=w1643:errorcluster)  [unwired: 8 in]
              n583 = property class="Clust (strict)"(reference=w1647, error in=w1643, "Value"=w1642) -> (error out=w1645:errorcluster)  [unwired: 1 out]
            }
            frame "Single Manip Jump" {
              n584 = Unbundle By Name(w1660) -> ("Single Manip Jump"=w1659:refnum<vi>)
              n585 = property class="Clust (strict)"(reference=w1659, error in=w1657) -> (reference out=w1658:refnum<vi>, error out=w1654:errorcluster, "Value"=w1652:T10)
              n586 = call "calc_singleManipJumpWaveform_v0.02.vi"("New input cluster"=w1652, "Clear Waveform?"=w1650, "Old input cluster"=w1652, "simulate Wave freq"=w1653, "error in"=w1654) -> ("output cluster"=w1651:T10, "error out"=w1655:errorcluster)  [unwired: 9 in]
              n587 = property class="Clust (strict)"(reference=w1658, error in=w1655, "Value"=w1651) -> (error out=w1656:errorcluster)  [unwired: 1 out]
            }
            frame "Multi M. Jump" {
              n588 = Unbundle By Name(w1671) -> ("Multi Manip Jump"=w1670:refnum<vi>)
              n589 = property class="Clust (strict)"(reference=w1670, error in=w1668) -> (reference out=w1669:refnum<vi>, error out=w1665:errorcluster, "Value"=w1663:T11)
              n590 = call "calc_multiManipJumpWaveform_v0.02.vi"("New input cluster"=w1663, "Clear Waveform?"=w1661, "Old input cluster"=w1663, "Numeric"=w1664, "error in"=w1665) -> ("output cluster"=w1662:T11, "error out"=w1666:errorcluster)  [unwired: 9 in]
              n591 = property class="Clust (strict)"(reference=w1669, error in=w1666, "Value"=w1662) -> (error out=w1667:errorcluster)  [unwired: 1 out]
            }
            frame "Voltage Pulse" {
              n592 = Unbundle By Name(w1682) -> ("Voltage Pulse"=w1681:refnum<vi>)
              n593 = property class="Clust (strict)"(reference=w1681, error in=w1679) -> (reference out=w1680:refnum<vi>, error out=w1676:errorcluster, "Value"=w1674:T12)
              n594 = call "calc_VoltagepulseWaveform_v0.03.vi"("New input cluster"=w1674, "Clear Waveform?"=w1672, "Old input cluster"=w1674, "sample freq"=w1675, "error in"=w1676) -> ("output cluster"=w1673:T12, "error out"=w1677:errorcluster)  [unwired: 9 in]
              n595 = property class="Clust (strict)"(reference=w1680, error in=w1677, "Value"=w1673) -> (error out=w1678:errorcluster)  [unwired: 1 out]
            }
            frame "Current Pulse" {
              n596 = Unbundle By Name(w1693) -> ("Current Pulse"=w1692:refnum<vi>)
              n597 = property class="Clust (strict)"(reference=w1692, error in=w1690) -> (reference out=w1691:refnum<vi>, error out=w1687:errorcluster, "Value"=w1685:T13)
              n598 = call "calc_CurrentpulseWaveform_v0.03.vi"("New input cluster"=w1685, "Clear Waveform?"=w1683, "Old input cluster"=w1685, "sample freq"=w1686, "error in"=w1687) -> ("output cluster"=w1684:T13, "error out"=w1688:errorcluster)  [unwired: 9 in]
              n599 = property class="Clust (strict)"(reference=w1691, error in=w1688, "Value"=w1684) -> (error out=w1689:errorcluster)  [unwired: 1 out]
            }
          }
        }
      }
      frame "PhaseL Cluster" {
        # "loop through all exp"
        n600 = Unbundle By Name(w1703) -> ("PhaseA Cluster"=w1702:T2)
        n601 = for {
          tunnel: w1702 -> [w1717]
          tunnel: w1701 -> [w1714] mode=indexing
          tunnel: w1700 -> [w1719]
          tunnel: [w1718] -> w1699
          tunnel: w1698 -> [w1707]
          tunnel: w1697 -> [w1713]
          tunnel: w1696 -> [w1712]
          tunnel: w1695 -> [w1711]
          tunnel: w1694 -> [w1710]
          n602 = Unbundle By Name(w1717) -> ("Phase Experiment Option"=w1716:refnum<vi>)
          n603 = property class="CmbBox"(reference=w1716) -> ("Value"=w1715:string)  [unwired: 1 in, 2 out]
          n604 = Equal?(x=w1715, y=w1714) -> (x = y?=w1708:bool)
          n605 = Greater?(x=w1711, y=w1710) -> (0:w1705:bool)
          n606 = Not(x=w1708) -> (.not. x?=w1709:bool)
          n607 = Select(t=w1707, s=w1707, f=w1709) -> (s? t:f=w1706:bool)
          n608 = Or(x=w1705, y=w1706) -> (x .or. y?=w1704:bool)
          n609 = case shown="\"Current Pulse\"" w1714 {
            tunnel: w1717 -> [w1731 w1743 w1754 w1765 w1776 w1787 w1799 w1810 w1821 w1832 w1843]
            tunnel: w1719 -> [w1727 w1740 w1751 w1762 w1773 w1784 w1796 w1807 w1818 w1829 w1840]
            tunnel: [w1724 w1739 w1750 w1761 w1772 w1783 w1795 w1806 w1817 w1828 w1839] -> w1718
            tunnel: w1713 -> [w1722 w1735 w1747 w1758 w1769 w1780 w1790 w1803 w1814 w1825 w1836]
            tunnel: w1712 -> [w1721 w1736 _ _ _ _ w1789 _ _ _ _]
            tunnel: w1704 -> [w1720 w1732 w1744 w1755 w1766 w1777 w1788 w1800 w1811 w1822 w1833]
            frame "Paired Pulse", Default {
              n610 = Unbundle By Name(w1731) -> ("Paired Pulse"=w1730:refnum<vi>)
              n611 = property class="Clust (strict)"(reference=w1730, error in=w1727) -> (reference out=w1728:refnum<vi>, error out=w1726:errorcluster, "Value"=w1729:T3)
              n612 = call "calc_PairedPulseWaveform_v0.02.vi"("New input cluster"=w1729, "Clear Waveform?"=w1720, "Old input cluster"=w1729, "Numeric"=w1722, "Jump Filter Freq (Hz)"=w1721, "error in"=w1726) -> ("output cluster"=w1723:T3, "error out"=w1725:errorcluster)  [unwired: 8 in]
              n613 = property class="Clust (strict)"(reference=w1728, error in=w1725, "Value"=w1723) -> (error out=w1724:errorcluster)  [unwired: 1 out]
            }
            frame "Jump Train" {
              n614 = Unbundle By Name(w1743) -> ("Jump Train"=w1742:refnum<vi>)
              n615 = property class="Clust (strict)"(reference=w1742, error in=w1740) -> (reference out=w1741:refnum<vi>, error out=w1738:errorcluster, "Value"=w1734:T4)
              n616 = call "calc_jumpTrainWaveform_v0.03.vi"("New input cluster"=w1734, "Clear Waveform?"=w1732, "Old input cluster"=w1734, "sample freq"=w1735, "Jump Filter Freq (Hz)"=w1736, "error in"=w1738) -> ("output cluster"=w1733:T4, "error out"=w1737:errorcluster)  [unwired: 8 in]
              n617 = property class="Clust (strict)"(reference=w1741, error in=w1737, "Value"=w1733) -> (error out=w1739:errorcluster)  [unwired: 1 out]
            }
            frame "Voltage Ramp" {
              n618 = Unbundle By Name(w1754) -> ("Voltage Ramp"=w1753:refnum<vi>)
              n619 = property class="Clust (strict)"(reference=w1753, error in=w1751) -> (reference out=w1752:refnum<vi>, error out=w1748:errorcluster, "Value"=w1746:T5)
              n620 = call "calc_VoltageRampWaveform_v0.03.vi"("New input cluster"=w1746, "Clear Waveform?"=w1744, "Old input cluster"=w1746, "sample freq"=w1747, "error in"=w1748) -> ("output cluster"=w1745:T5, "error out"=w1749:errorcluster)  [unwired: 9 in]
              n621 = property class="Clust (strict)"(reference=w1752, error in=w1749, "Value"=w1745) -> (error out=w1750:errorcluster)  [unwired: 1 out]
            }
            frame "Current Ramp" {
              n622 = Unbundle By Name(w1765) -> ("Current Ramp"=w1764:refnum<vi>)
              n623 = property class="Clust (strict)"(reference=w1764, error in=w1762) -> (reference out=w1763:refnum<vi>, error out=w1759:errorcluster, "Value"=w1757:T6)
              n624 = call "calc_CurrentRampWaveform_v0.03.vi"("New input cluster"=w1757, "Clear Waveform?"=w1755, "Old input cluster"=w1757, "sample freq"=w1758, "error in"=w1759) -> ("output cluster"=w1756:T6, "error out"=w1760:errorcluster)  [unwired: 9 in]
              n625 = property class="Clust (strict)"(reference=w1763, error in=w1760, "Value"=w1756) -> (error out=w1761:errorcluster)  [unwired: 1 out]
            }
            frame "Voltage Step" {
              n626 = Unbundle By Name(w1776) -> ("Voltage Step"=w1775:refnum<vi>)
              n627 = property class="Clust (strict)"(reference=w1775, error in=w1773) -> (reference out=w1774:refnum<vi>, error out=w1770:errorcluster, "Value"=w1768:T7)
              n628 = call "calc_VoltageStepWaveform_v0.03.vi"("New input cluster"=w1768, "Clear Waveform?"=w1766, "Old input cluster"=w1768, "sample freq"=w1769, "error in"=w1770) -> ("output cluster"=w1767:T7, "error out"=w1771:errorcluster)  [unwired: 9 in]
              n629 = property class="Clust (strict)"(reference=w1774, error in=w1771, "Value"=w1767) -> (error out=w1772:errorcluster)  [unwired: 1 out]
            }
            frame "Solution Change" {
              n630 = Unbundle By Name(w1787) -> ("Solution Change"=w1786:refnum<vi>)
              n631 = property class="Clust (strict)"(reference=w1786, error in=w1784) -> (reference out=w1785:refnum<vi>, error out=w1781:errorcluster, "Value"=w1779:T8)
              n632 = call "calc_SolutionChangeWaveform_v0.03.vi"("New input cluster"=w1779, "Clear Waveform?"=w1777, "Old input cluster"=w1779, "sample freq"=w1780, "error in"=w1781) -> ("output cluster"=w1778:T8, "error out"=w1782:errorcluster)  [unwired: 9 in]
              n633 = property class="Clust (strict)"(reference=w1785, error in=w1782, "Value"=w1778) -> (error out=w1783:errorcluster)  [unwired: 1 out]
            }
            frame "Single Jump" {
              n634 = Unbundle By Name(w1799) -> ("Single Jump"=w1798:refnum<vi>)
              n635 = property class="Clust (strict)"(reference=w1798, error in=w1796) -> (reference out=w1797:refnum<vi>, error out=w1794:errorcluster, "Value"=w1791:T9)
              n636 = call "calc_sinlge JumpWaveform_v0.03.vi"("New input cluster"=w1791, "Clear Waveform?"=w1788, "Old input cluster"=w1791, "sample freq"=w1790, "Jump Filter Freq (Hz)"=w1789, "error in"=w1794) -> ("output cluster"=w1792:T9, "error out"=w1793:errorcluster)  [unwired: 8 in]
              n637 = property class="Clust (strict)"(reference=w1797, error in=w1793, "Value"=w1792) -> (error out=w1795:errorcluster)  [unwired: 1 out]
            }
            frame "Single Manip Jump" {
              n638 = Unbundle By Name(w1810) -> ("Single Manip Jump"=w1809:refnum<vi>)
              n639 = property class="Clust (strict)"(reference=w1809, error in=w1807) -> (reference out=w1808:refnum<vi>, error out=w1804:errorcluster, "Value"=w1802:T10)
              n640 = call "calc_singleManipJumpWaveform_v0.02.vi"("New input cluster"=w1802, "Clear Waveform?"=w1800, "Old input cluster"=w1802, "simulate Wave freq"=w1803, "error in"=w1804) -> ("output cluster"=w1801:T10, "error out"=w1805:errorcluster)  [unwired: 9 in]
              n641 = property class="Clust (strict)"(reference=w1808, error in=w1805, "Value"=w1801) -> (error out=w1806:errorcluster)  [unwired: 1 out]
            }
            frame "Multi M. Jump" {
              n642 = Unbundle By Name(w1821) -> ("Multi Manip Jump"=w1820:refnum<vi>)
              n643 = property class="Clust (strict)"(reference=w1820, error in=w1818) -> (reference out=w1819:refnum<vi>, error out=w1815:errorcluster, "Value"=w1813:T11)
              n644 = call "calc_multiManipJumpWaveform_v0.02.vi"("New input cluster"=w1813, "Clear Waveform?"=w1811, "Old input cluster"=w1813, "Numeric"=w1814, "error in"=w1815) -> ("output cluster"=w1812:T11, "error out"=w1816:errorcluster)  [unwired: 9 in]
              n645 = property class="Clust (strict)"(reference=w1819, error in=w1816, "Value"=w1812) -> (error out=w1817:errorcluster)  [unwired: 1 out]
            }
            frame "Voltage Pulse" {
              n646 = Unbundle By Name(w1832) -> ("Voltage Pulse"=w1831:refnum<vi>)
              n647 = property class="Clust (strict)"(reference=w1831, error in=w1829) -> (reference out=w1830:refnum<vi>, error out=w1826:errorcluster, "Value"=w1824:T12)
              n648 = call "calc_VoltagepulseWaveform_v0.03.vi"("New input cluster"=w1824, "Clear Waveform?"=w1822, "Old input cluster"=w1824, "sample freq"=w1825, "error in"=w1826) -> ("output cluster"=w1823:T12, "error out"=w1827:errorcluster)  [unwired: 9 in]
              n649 = property class="Clust (strict)"(reference=w1830, error in=w1827, "Value"=w1823) -> (error out=w1828:errorcluster)  [unwired: 1 out]
            }
            frame "Current Pulse" {
              n650 = Unbundle By Name(w1843) -> ("Current Pulse"=w1842:refnum<vi>)
              n651 = property class="Clust (strict)"(reference=w1842, error in=w1840) -> (reference out=w1841:refnum<vi>, error out=w1837:errorcluster, "Value"=w1835:T13)
              n652 = call "calc_CurrentpulseWaveform_v0.03.vi"("New input cluster"=w1835, "Clear Waveform?"=w1833, "Old input cluster"=w1835, "sample freq"=w1836, "error in"=w1837) -> ("output cluster"=w1834:T13, "error out"=w1838:errorcluster)  [unwired: 9 in]
              n653 = property class="Clust (strict)"(reference=w1841, error in=w1838, "Value"=w1834) -> (error out=w1839:errorcluster)  [unwired: 1 out]
            }
          }
        }
      }
    }
  }
  "error out" <- w7
